vi "PC MAIN.vi"() -> ()   [LabVIEW 2017]
uses:
  <vilib>/Platform/TimedLoop/XDataNode/timing_clust.ctl
  <vilib>/Platform/TimedLoop/XDataNode/nitl_modes.ctl
  <vilib>/Platform/TimedLoop/XDataNode/wakeup.ctl
  <vilib>/imath/engines/lvmath2/RunTimeEngine/IndexRead/NIMS V(S).vi
  <instcachedir>/0/NIMS V(S)_0488751826AF41519A22953C041130DC.lvgen/NIMS V(S)_0488751826AF41519A22953C041130DC_000.vi
  <vilib>/imathl/engines/lvmath/Functions/Error Handling/Create Error.vi
  <vilib>/imath/engines/lvmath2/RunTimeEngine/BuiltInFunctions/atan2/NIMS_atan2.vi
  <instcachedir>/0/NIMS_atan2_A91AA4A7D42247EDBE8F76DB99AF04A4.lvgen/NIMS_atan2_A91AA4A7D42247EDBE8F76DB99AF04A4_000.vi
  <vilib>/imath/engines/lvmath2/RunTimeEngine/IndexReplace/NIMS V(S)=S.vi
  <instcachedir>/0/NIMS V(S)=S_3F4D177D41884A9C969E5FA0B22E4B28.lvgen/NIMS V(S)=S_3F4D177D41884A9C969E5FA0B22E4B28_000.vi
  <vilib>/imath/engines/lvmath2/RunTimeEngine/ArithmeticOperatorToken/NIMS_ArithmeticOperator_power(S).vi
  <instcachedir>/0/NIMS_ArithmeticOperator_power(S)_86B1D76B77564424912EAFCCCC7488ED.lvgen/NIMS_ArithmeticOperator_power(S)_86B1D76B77564424912EAFCCCC7488ED_010.vi
  <vilib>/imath/engines/lvmath2/RunTimeEngine/BuiltInFunctions/acos/NIMS_acos(C).vi
  <instcachedir>/0/NIMS_acos(C)_09AB0EA1D77D44F8AD620F57E6E2841E.lvgen/NIMS_acos(C)_09AB0EA1D77D44F8AD620F57E6E2841E_001.vi
  <instcachedir>/0/NIMS_atan2_A91AA4A7D42247EDBE8F76DB99AF04A4.lvgen/NIMS_atan2_A91AA4A7D42247EDBE8F76DB99AF04A4_001.vi
  <vilib>/imath/engines/lvmath2/RunTimeEngine/BuiltInFunctions/asin/NIMS_asin(C).vi
  <instcachedir>/0/NIMS_asin(C)_AC3BFCB47B1546A49EF59786BF54013C.lvgen/NIMS_asin(C)_AC3BFCB47B1546A49EF59786BF54013C_001.vi
  <instcachedir>/0/NIMS V(S)=S_3F4D177D41884A9C969E5FA0B22E4B28.lvgen/NIMS V(S)=S_3F4D177D41884A9C969E5FA0B22E4B28_001.vi
  <vilib>/imath/engines/lvmath2/RunTimeEngine/ErrorHandling/NIMS_Create Error From Enums.vi
  <instcachedir>/0/NIMS V(S)_0488751826AF41519A22953C041130DC.lvgen/NIMS V(S)_0488751826AF41519A22953C041130DC_003.vi
  <vilib>/imath/engines/lvmath2/RunTimeEngine/BuiltInFunctions/sin/NIMS_sin(C).vi
  <instcachedir>/0/NIMS_sin(C)_3AEF00A0D47841AA8A3F5FC7392BEEFD.lvgen/NIMS_sin(C)_3AEF00A0D47841AA8A3F5FC7392BEEFD_001.vi
  <vilib>/imath/engines/lvmath2/RunTimeEngine/BuiltInFunctions/cos/NIMS_cos(C).vi
  <instcachedir>/0/NIMS_cos(C)_D76AB42705D04DD7AB90183D51B32C21.lvgen/NIMS_cos(C)_D76AB42705D04DD7AB90183D51B32C21_001.vi
  <vilib>/imath/engines/lvmath2/RunTimeEngine/BuiltInFunctions/pinv/NIMS_pinv.vi
  <instcachedir>/0/NIMS_pinv_206F0700CF75499C820074BA4F1FFC36.lvgen/NIMS_pinv_206F0700CF75499C820074BA4F1FFC36_001.vi
  <vilib>/imath/engines/lvmath2/RunTimeEngine/ArithmeticOperatorToken/NIMS_ArithmeticOperator_multmx(M,CV).vi
  <instcachedir>/0/NIMS_ArithmeticOperator_multmx(M,CV)_C4CEBAC88ACD4FCE9121CEED56911FC5.lvgen/NIMS_ArithmeticOperator_multmx(M,CV)_C4CEBAC88ACD4FCE9121CEED56911FC5_002.vi
  <vilib>/imath/engines/lvmath2/RunTimeEngine/IndexRead/NIMS M($,S).vi
  <instcachedir>/0/NIMS M($,S)_3E5749BBB62E49528D4765A77F1F6D98.lvgen/NIMS M($,S)_3E5749BBB62E49528D4765A77F1F6D98_001.vi
  <vilib>/imath/engines/lvmath2/RunTimeEngine/NodeEndStatement/NIMS_NodeEndStatement_Output.vi
  <instcachedir>/0/NIMS_NodeEndStatement_Output_53EC0D466D134D7ABD903AC30B43404B.lvgen/NIMS_NodeEndStatement_Output_53EC0D466D134D7ABD903AC30B43404B_000.vi
  <vilib>/imath/engines/lvmath2/RunTimeEngine/ErrorHandling/NIMS_Finalize Error.vi
  <vilib>/imath/engines/lvmath2/RunTimeEngine/RangeToken/NIMS_Range_R2 - Integer.vi
  <instcachedir>/0/NIMS_Range_R2 - Integer_B2C3C6B11D0E4F789E1772ACB483EB02.lvgen/NIMS_Range_R2 - Integer_B2C3C6B11D0E4F789E1772ACB483EB02_000.vi
  <vilib>/imath/engines/lvmath2/RunTimeEngine/CommandStatement/MC_CommandStatement_break.vi
  <vilib>/imath/engines/lvmath2/RunTimeEngine/VariableToken/NIMS_VariableToken_CondDefinedDefinedByReplace.vi
  <instcachedir>/0/NIMS_VariableToken_CondDefinedDefinedByReplace_D162CFFC24174562A9FEA619A91E1A56.lvgen/NIMS_VariableToken_CondDefinedDefinedByReplace_D162CFFC24174562A9FEA619A91E1A56_000.vi
  <instcachedir>/0/NIMS_VariableToken_CondDefinedDefinedByReplace_D162CFFC24174562A9FEA619A91E1A56.lvgen/NIMS_VariableToken_CondDefinedDefinedByReplace_D162CFFC24174562A9FEA619A91E1A56_003.vi
  <instcachedir>/0/NIMS_VariableToken_CondDefinedDefinedByReplace_D162CFFC24174562A9FEA619A91E1A56.lvgen/NIMS_VariableToken_CondDefinedDefinedByReplace_D162CFFC24174562A9FEA619A91E1A56_002.vi
  <vilib>/imath/engines/lvmath2/RunTimeEngine/VariableToken/NIMS_VariableToken_CondDefined.vi
  <instcachedir>/0/NIMS_VariableToken_CondDefined_6E7F1EE7F80E48298C84CF05BD736261.lvgen/NIMS_VariableToken_CondDefined_6E7F1EE7F80E48298C84CF05BD736261_000.vi
  <vilib>/imath/engines/lvmath2/RunTimeEngine/IndexReplace/NIMS M(S,S)=S.vi
  <instcachedir>/0/NIMS M(S,S)=S_490F2BBDD0204024B81939EC402D9A55.lvgen/NIMS M(S,S)=S_490F2BBDD0204024B81939EC402D9A55_001.vi
  <instcachedir>/0/NIMS_VariableToken_CondDefined_6E7F1EE7F80E48298C84CF05BD736261.lvgen/NIMS_VariableToken_CondDefined_6E7F1EE7F80E48298C84CF05BD736261_002.vi
  <instcachedir>/0/NIMS_NodeEndStatement_Output_53EC0D466D134D7ABD903AC30B43404B.lvgen/NIMS_NodeEndStatement_Output_53EC0D466D134D7ABD903AC30B43404B_003.vi
  <vilib>/platform/TimedLoop/XDataNode/XDataNode.xnode
  <vilib>/Platform/TimedLoop/XDataNode/XDNodeRunTimeDep.lvlib
panel:
  in  "Z-":bool
  in  "Z+":bool
  in  "Y-":bool
  in  "Y+":bool
  in  "X-":bool
  out "x":dbl[][](array[numeric])
  in  "Increment(0-10mm)":dbl min=-10.0 max=10.0 step=1.0
  in  "X+":bool
  out "Joint3":dbl
  out "Joint2":dbl
  out "Joint1":dbl
  in  "Circle":bool
  out "circle":dbl[](array[numeric])
  out "line":dbl[](array[numeric])
  in  "Line":bool
  in  "DIR3":bool
  in  "Duty cycle3":dbl
  in  "Frequency3":dbl
  in  "DIR2":bool
  in  "Duty cycle2":dbl
  in  "Frequency2":dbl
  in  "RT STOP":bool
  in  "DIR1":bool
  in  "Duty cycle1":dbl
  in  "Frequency1":dbl
  in  "STOP":bool
  # "Motor Status"
  # "Control Pad"
  # "Joint Angle(Deg)"
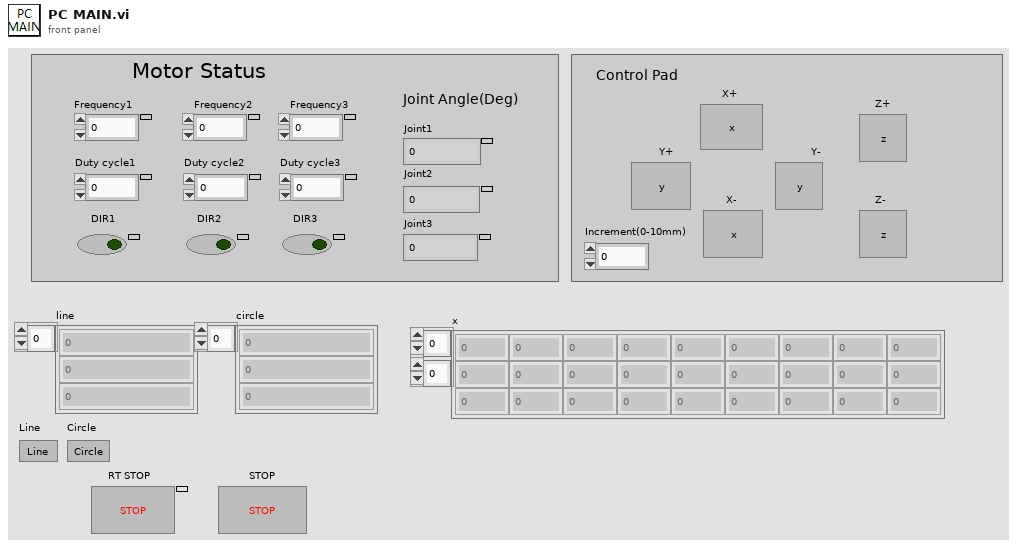
[diagram p1: front panel]
types:
  T1 = typedef "XDNodeRunTimeDep.lvlib/timing_clust.ctl" = cluster{"Expected End [f-1]":u64, "Actual End [f-1]":u64, "Finished Late? [f-1]":bool, "Expected End [i-1]":u64, "Actual End [i-1]":u64, "Finished Late? [i-1]":bool, "Expected Start [i]":u64, "Actual Start [i]":u64, "Expected Start [f]":u64, "Actual Start [f]":u64, "Source Name":string, "Structure Name":string, "Period":i64, "Deadline":i64, "Offset":i64, "Start":i64, "Priority":i32, "Timeout":i32, "Mode":T2, "Wakeup Reason":T3, "Error":errorcluster, "Source Type":string, "Secondary Source Type":string, "Global End Time":u64, "Global Start Time":u64, "Frame Duration":u64, "Iteration Duration":u64, "Assigned CPU":i32, "I/O Scan Engine Mode":u32}
  T2 = typedef "XDNodeRunTimeDep.lvlib/nitl_modes.ctl" = enum32{"No Change", "Process missed periods, maintain original phase", "Discard missed periods, maintain original phase", "Process missed periods, ignore original phase", "Discard missed periods, ignore original phase"}
  T3 = typedef "XDNodeRunTimeDep.lvlib/wakeup.ctl" = enum32{"Normal", "Aborted", "Asynchronous wakeup", "Timing source error", "Timed loop error", "Timeout"}
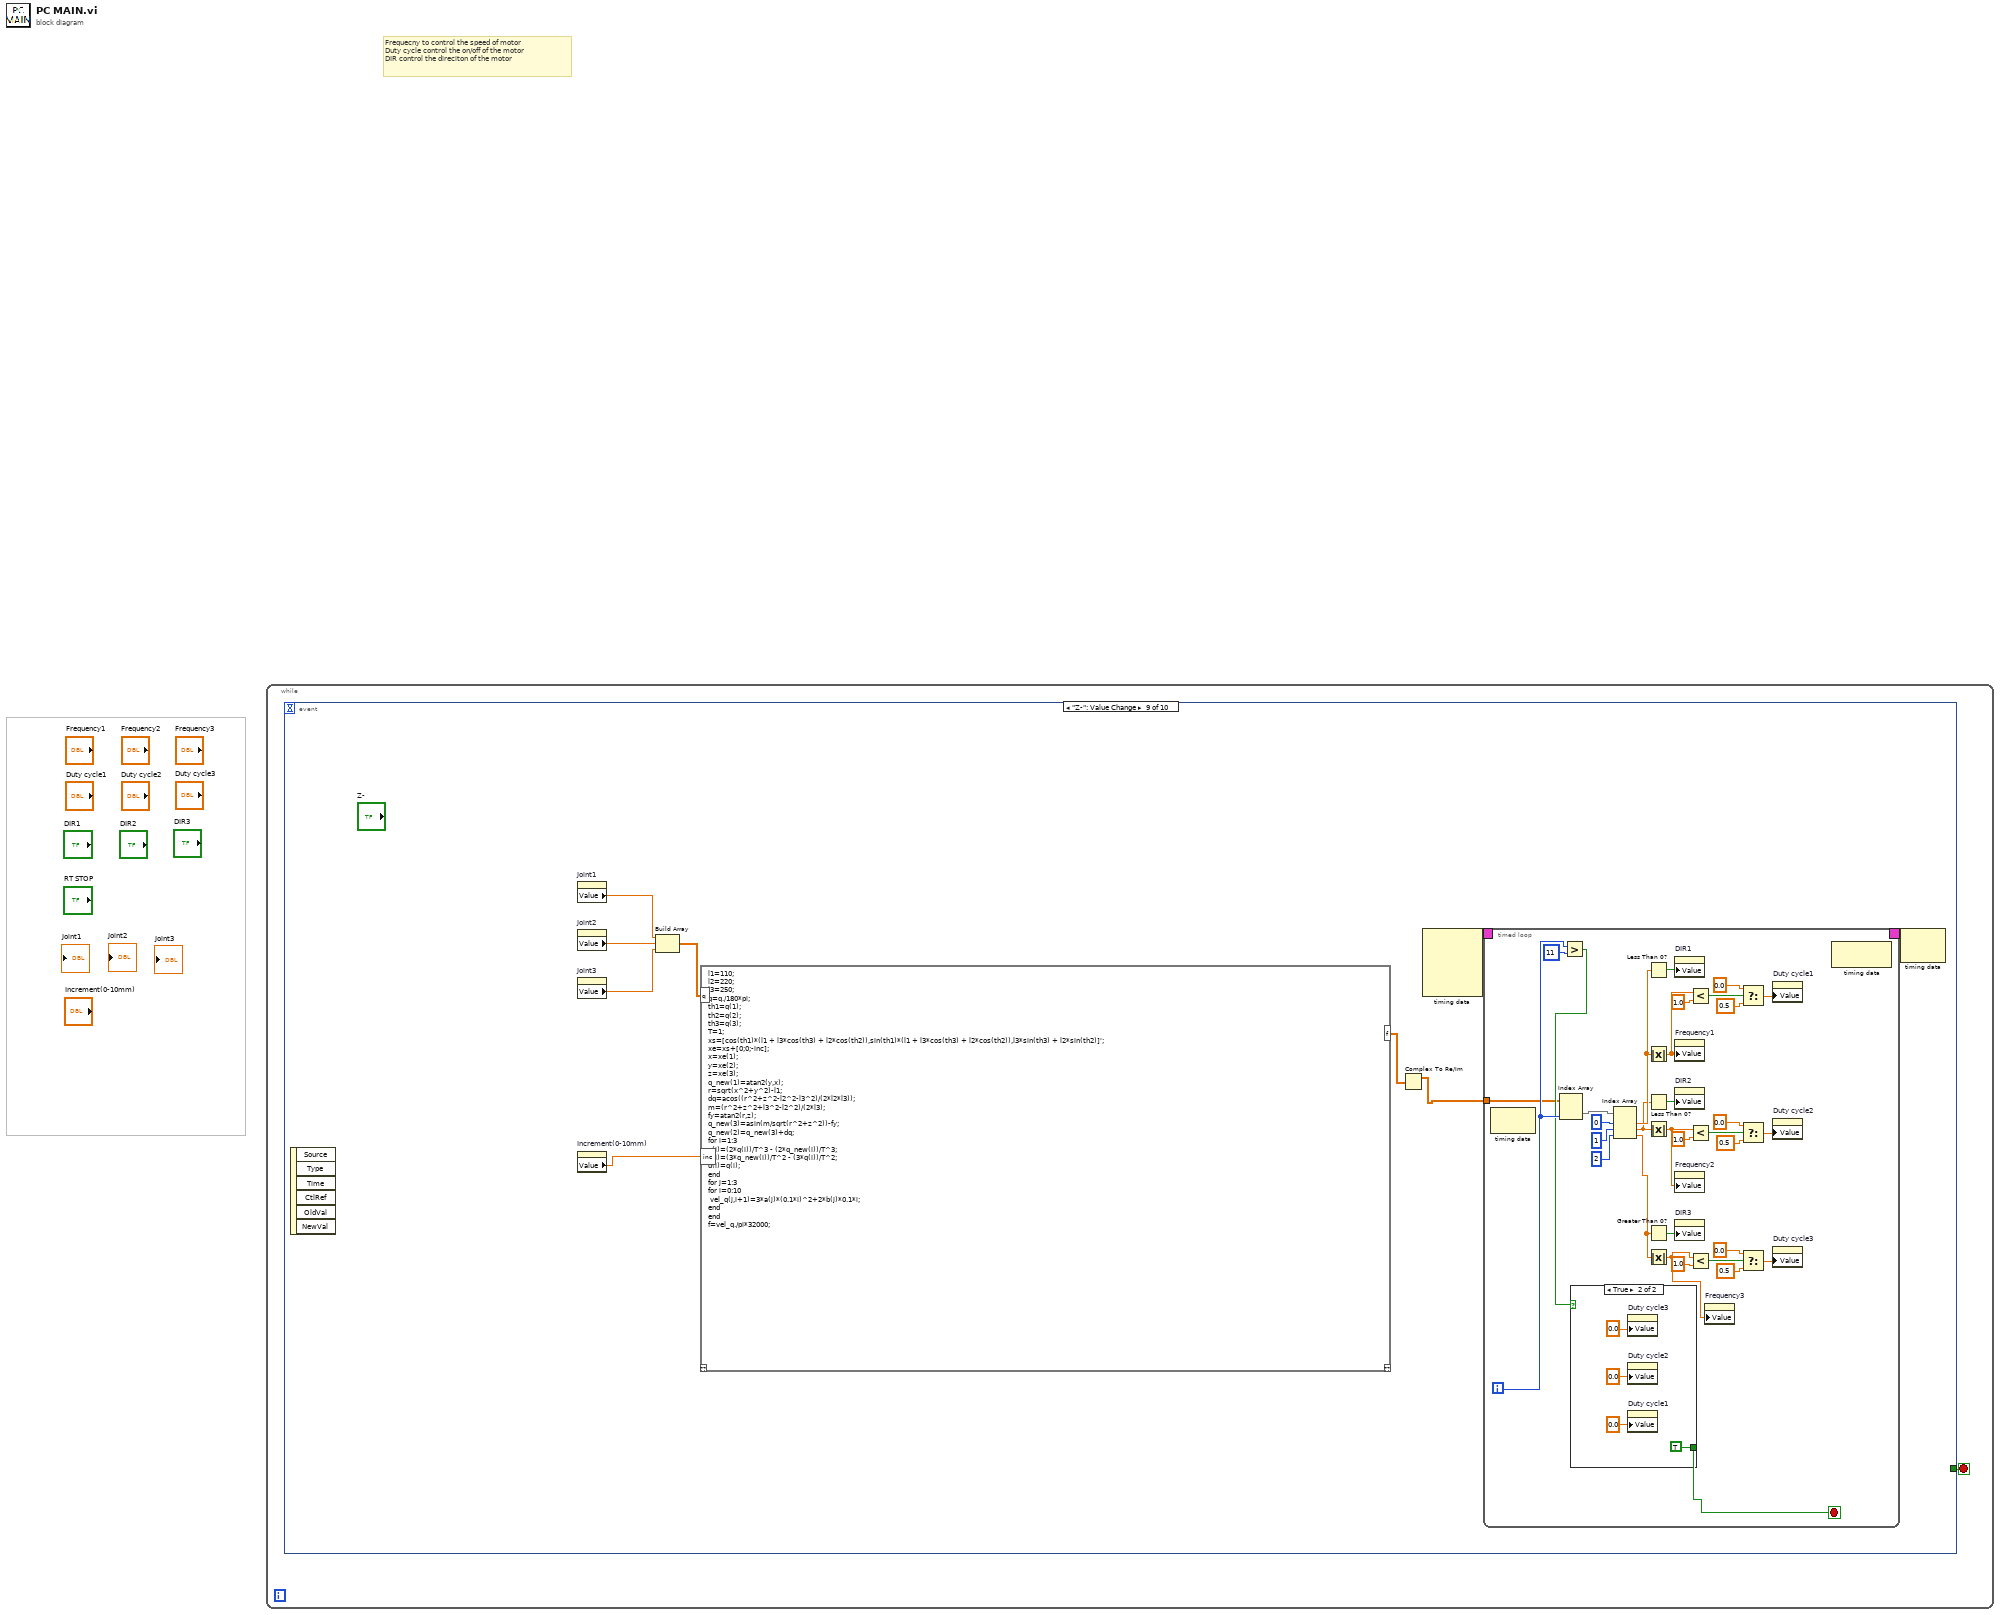
[diagram p0: block diagram]
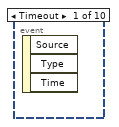
[diagram p2: hidden frame]
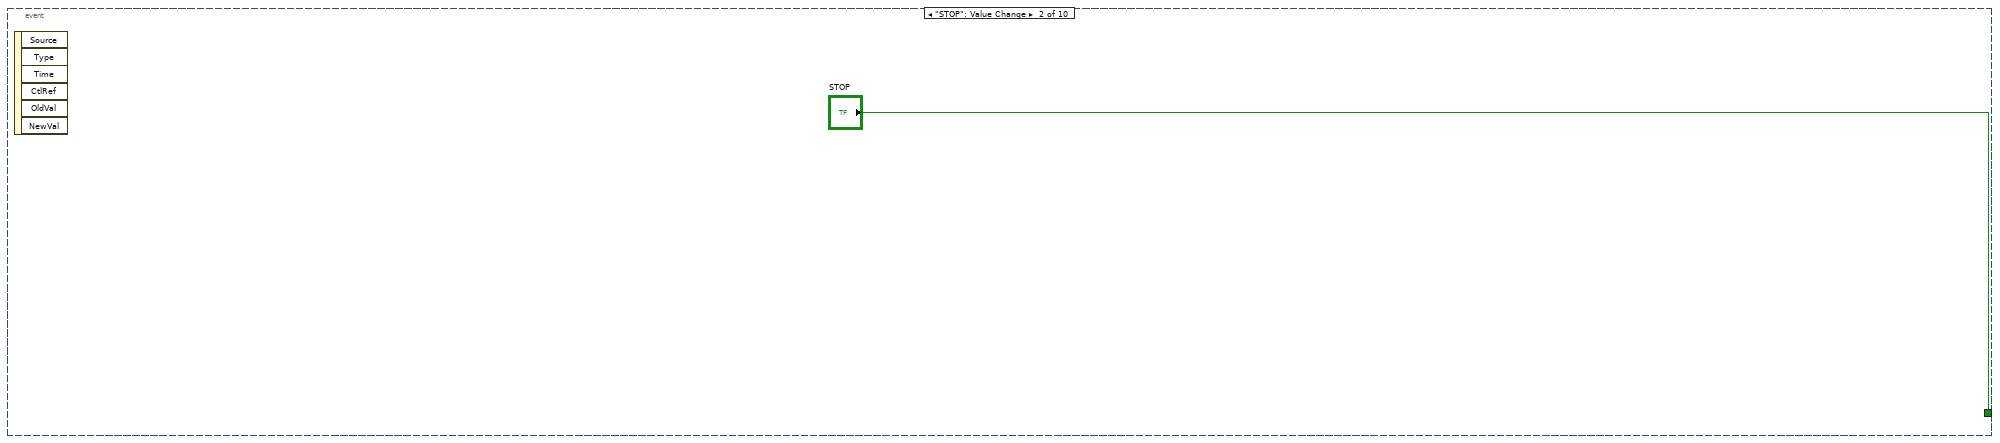
[diagram p3: hidden frame]
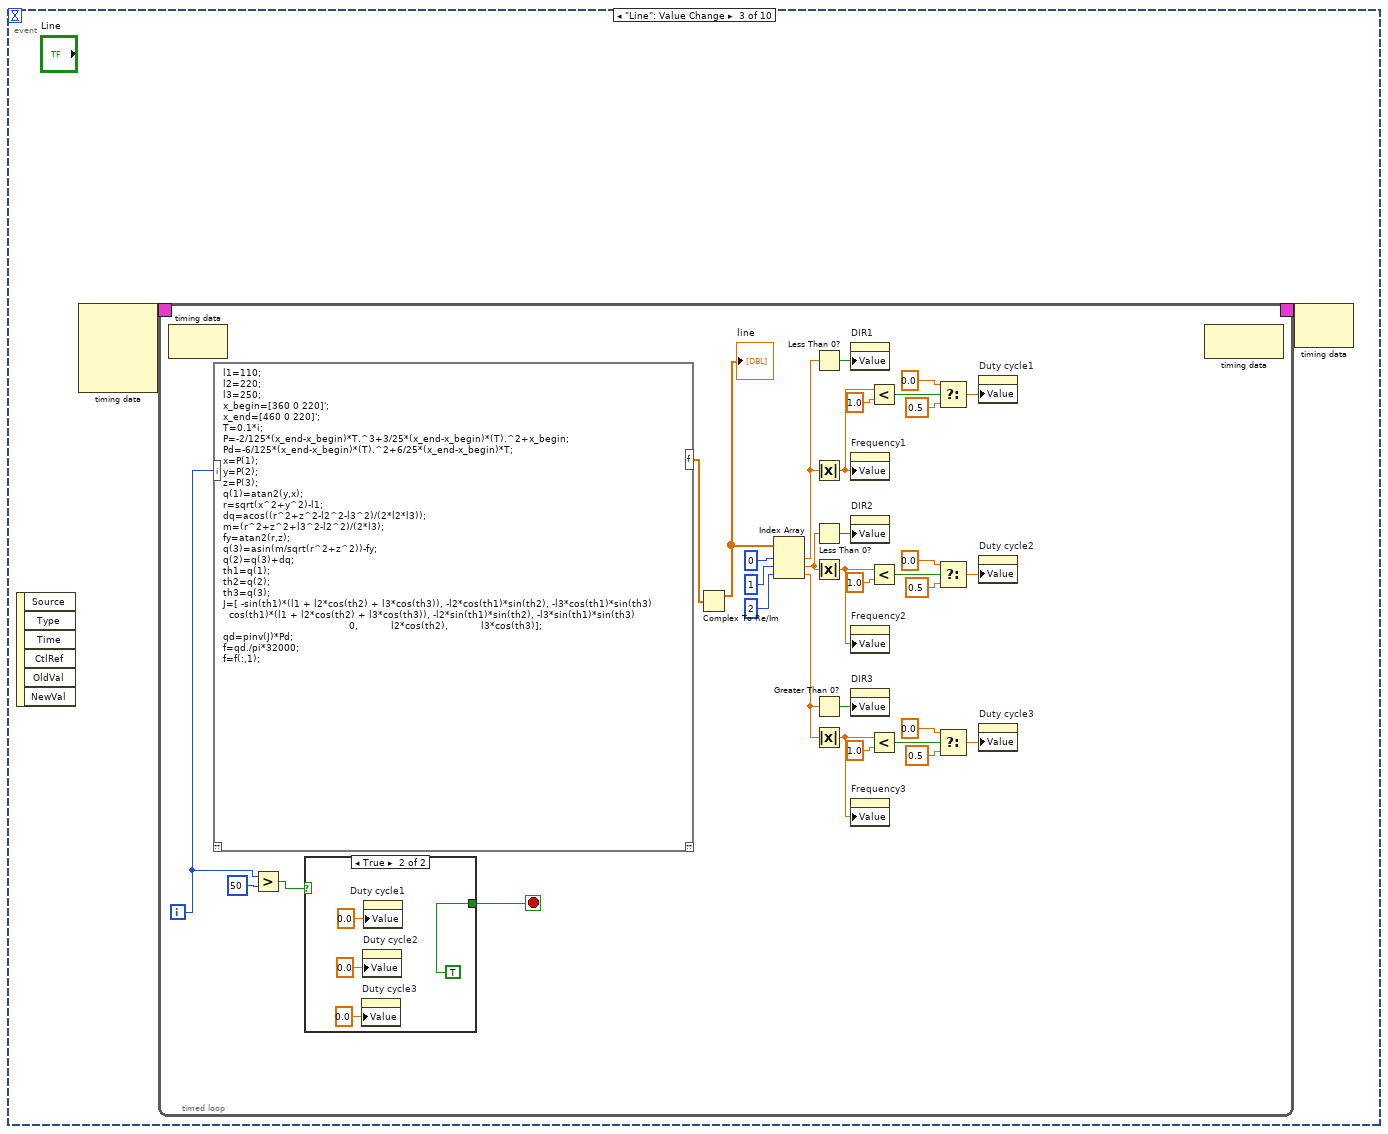
[diagram p4: hidden frame]
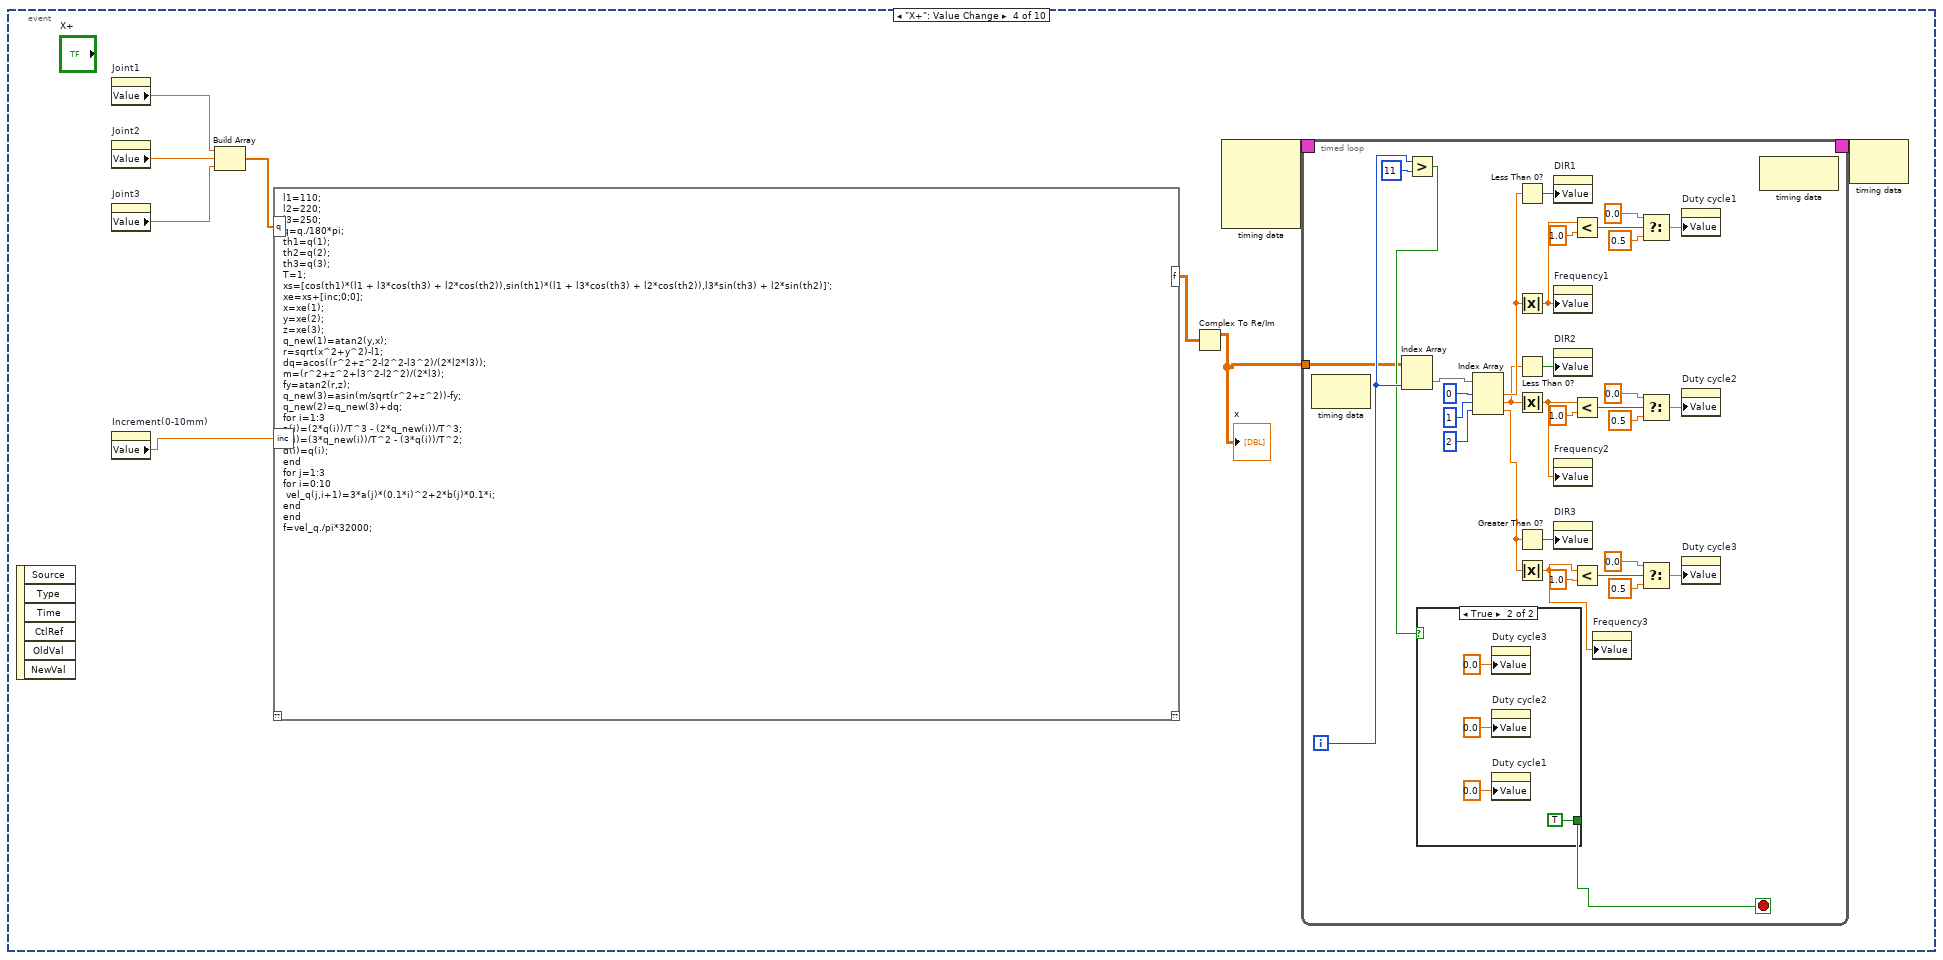
[diagram p6: hidden frame]
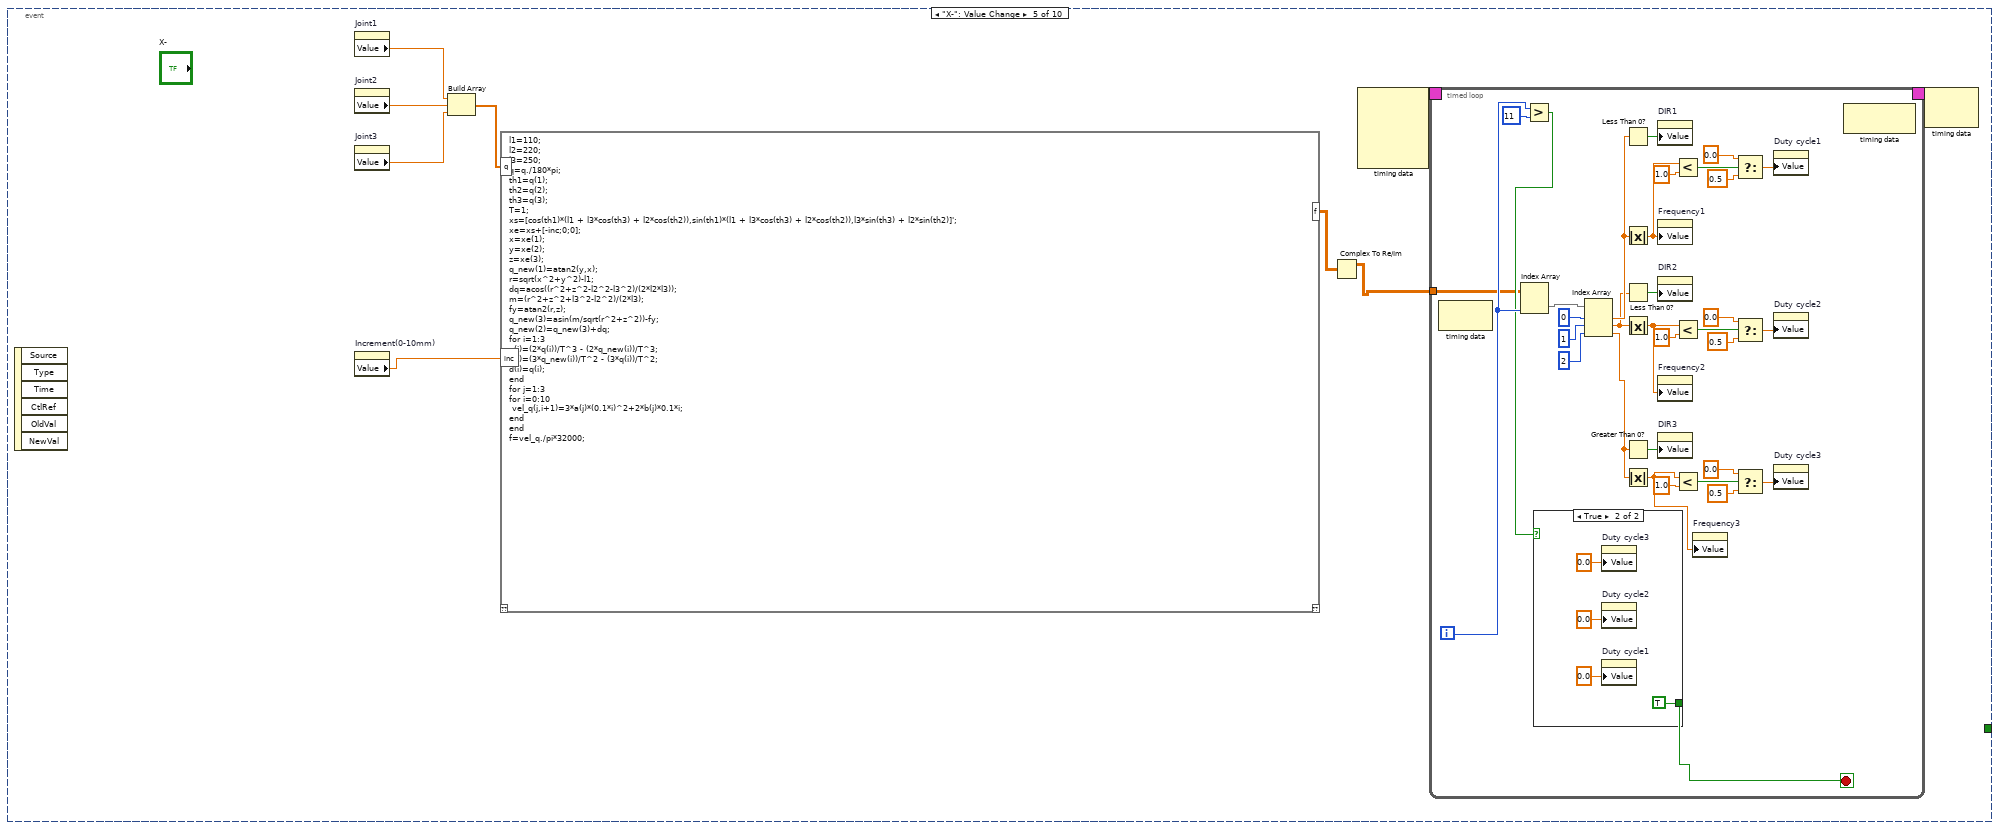
[diagram p8: hidden frame]
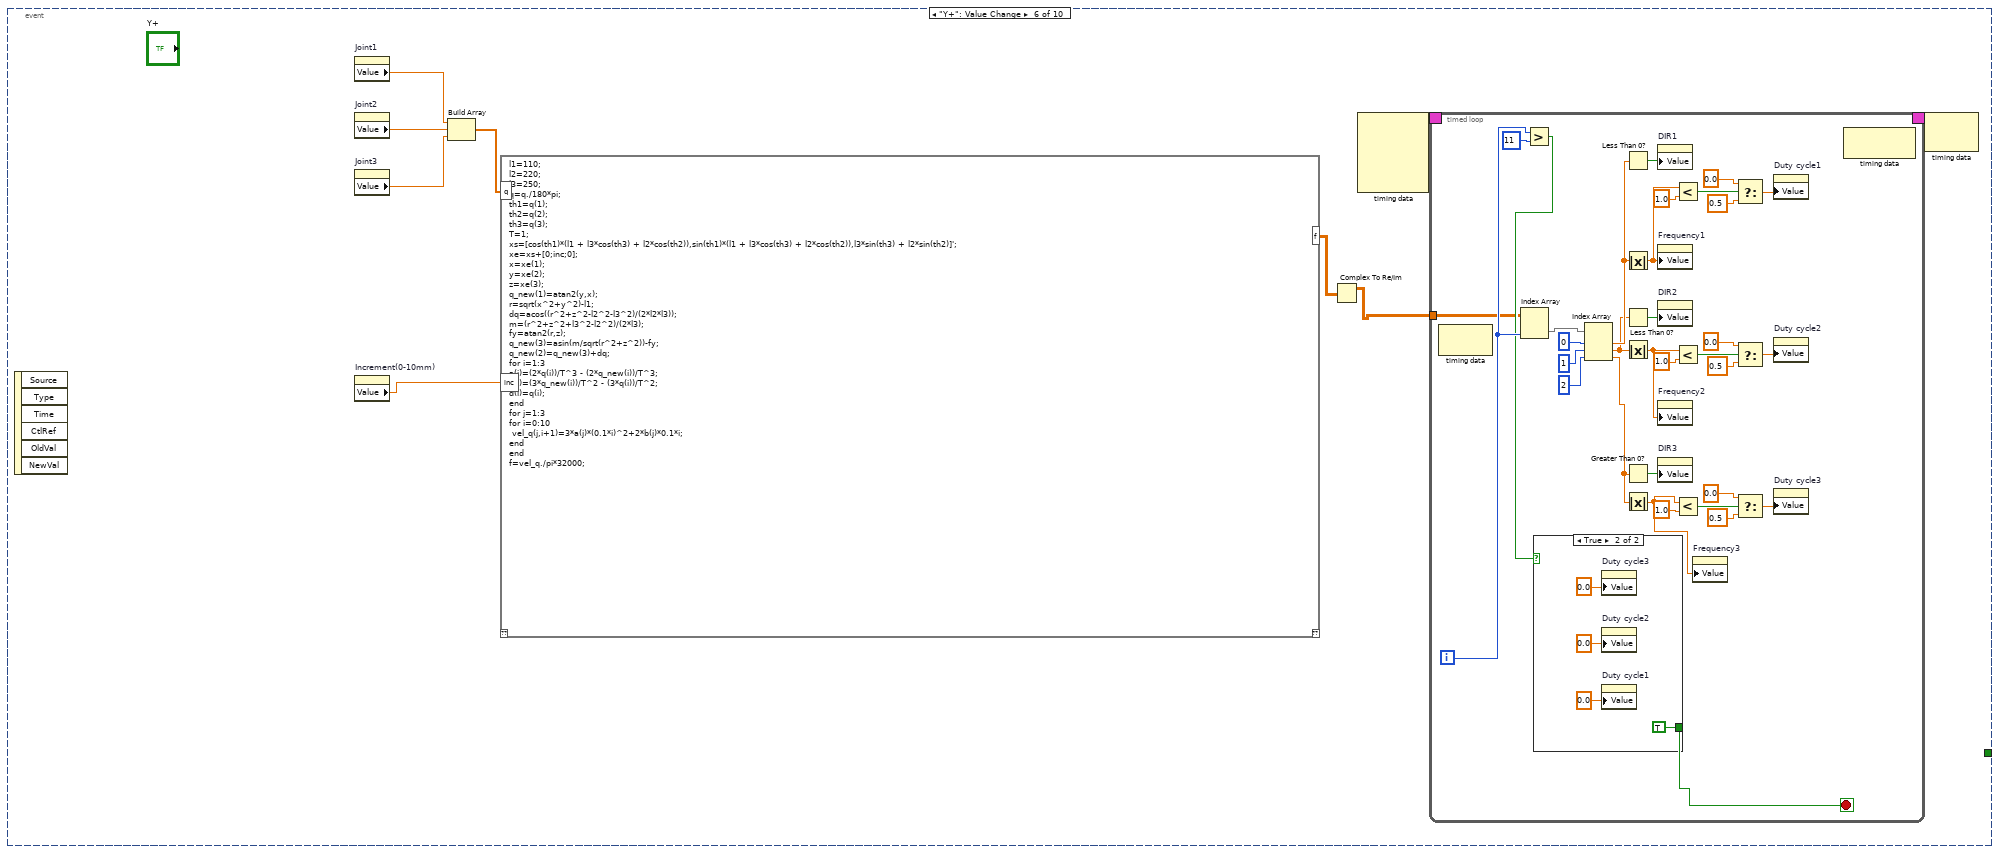
[diagram p10: hidden frame]
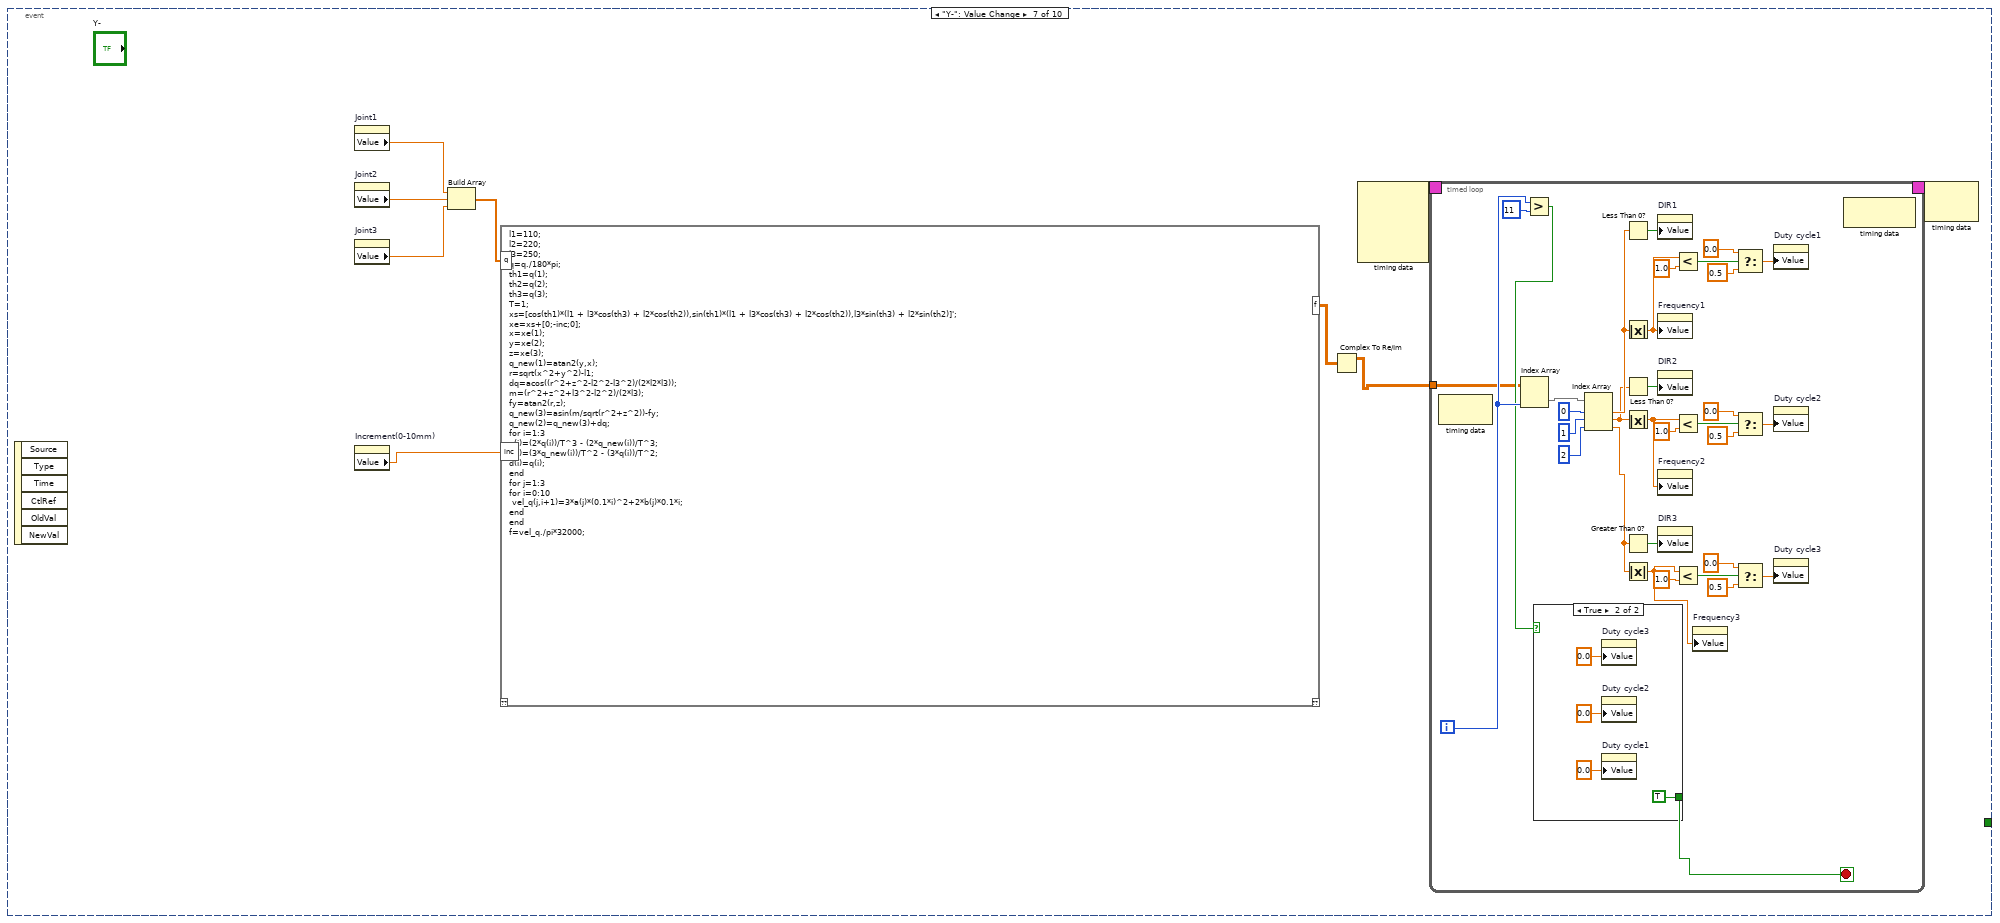
[diagram p12: hidden frame]
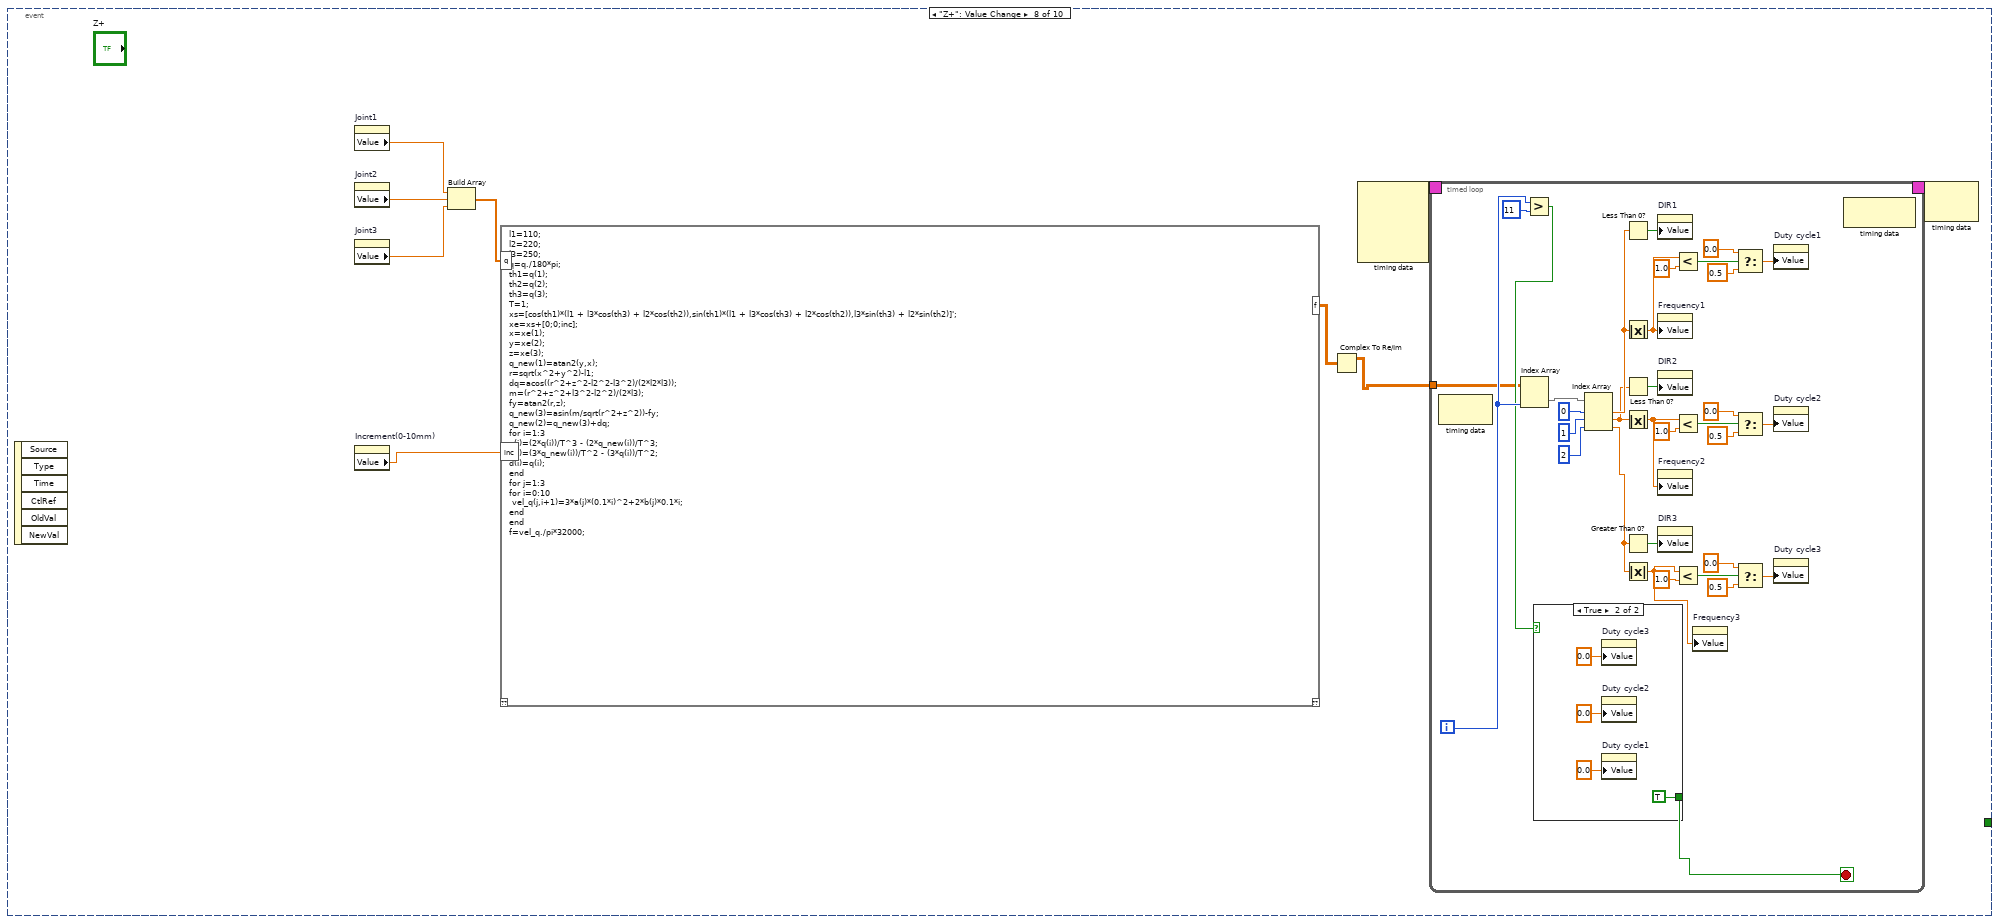
[diagram p14: hidden frame]
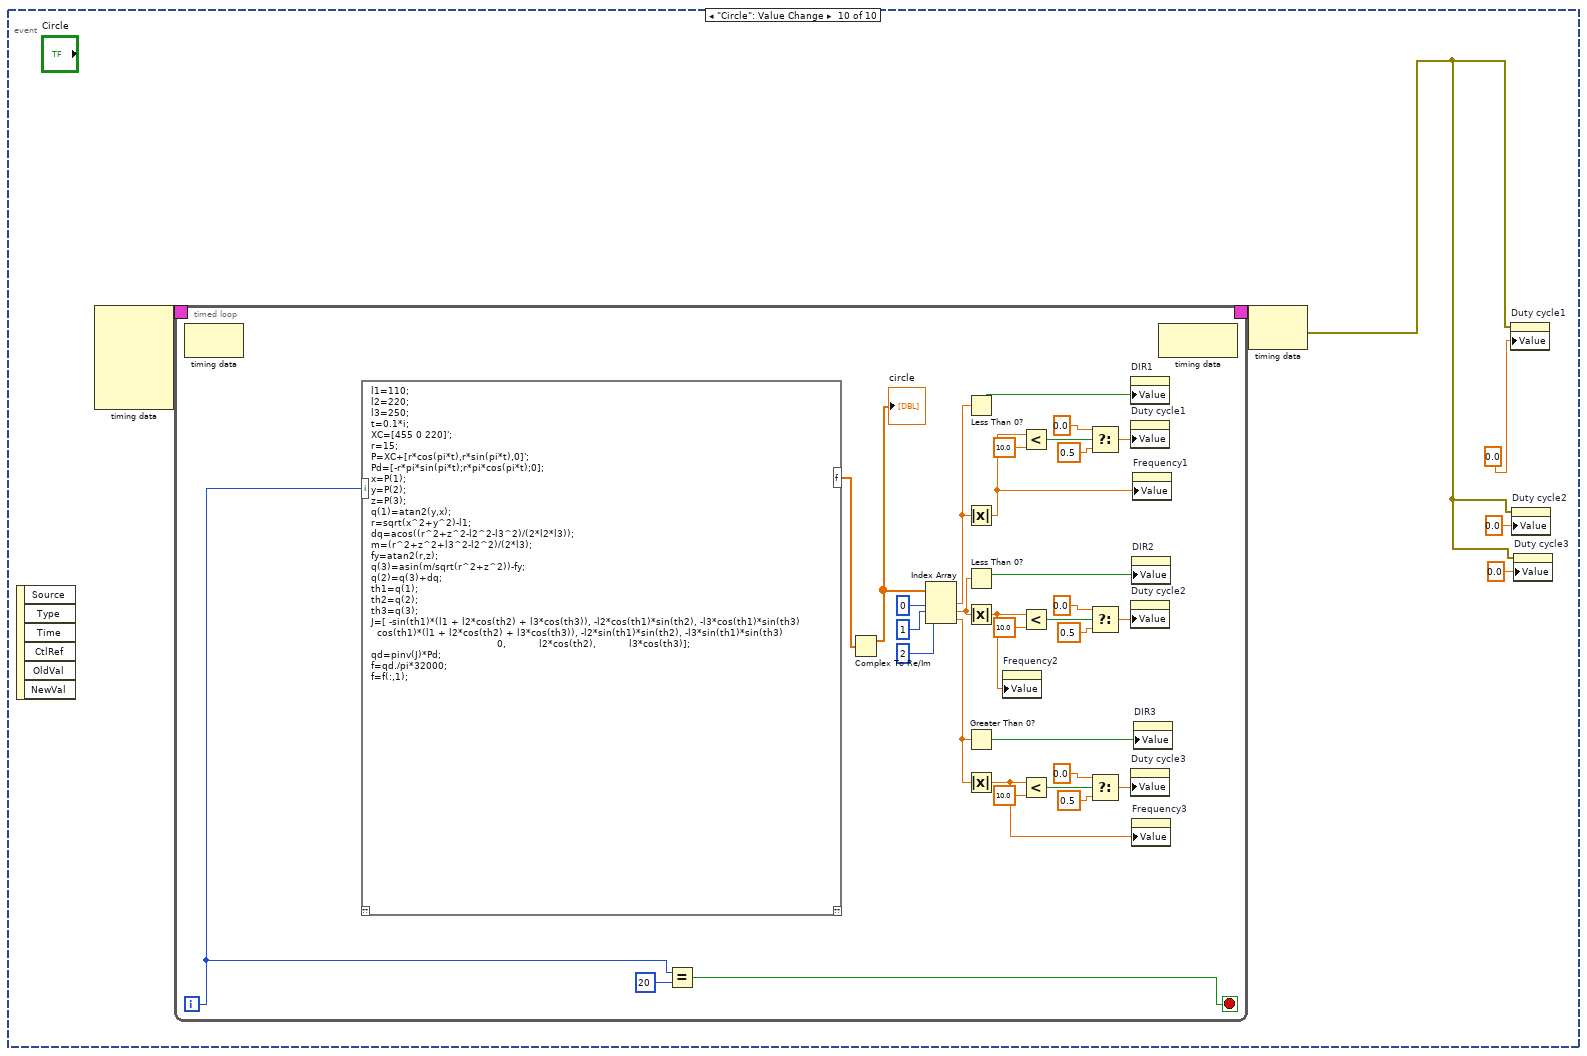
[diagram p17: hidden frame]
diagram:
  # "Frequecny to control the speed of motor \nDuty cycle control the on/off of the motor\nDIR control the direciton of the motor"
  n1 = while {
    stop <- w1 stop-if-true
    n2 = event shown="[8] \"Z-\": Value Change" {
      selector: _ -> [_ _ _ _ _ _ _ _ _ _]
      dyn-events: _ -> [_ _ _ _ _ _ _ _ _ _]
      timeout: _ -> [_ _ _ _ _ _ _ _ _ _]
      tunnel: [_ "STOP" _ _ _ _ _ _ _ _] -> w1
      event Timeout {
        n3 = event-data() -> ()  [unwired: 1 in, 3 out]
      }
      event "STOP": Value Change {
        n4 = event-data() -> ()  [unwired: 1 in, 6 out]
      }
      event "Line": Value Change {
        n5 = event-data() -> ()  [unwired: 1 in, 6 out]
        n6 = node-c288() -> (w4:T1)  [unwired: 4 in]
        n7 = timed-loop {
          timing: w4 -> [_]
          timing-out: [_] -> w3
          i -> [w37]
          stop <- w5 stop-if-true
          n8 = node-c288() -> ()  [unwired: 1 in, 1 out]
          n9 = mathscript code="l1=110;\nl2=220;\nl3=250;\nx_begin=[360 0 220]';\nx_end=[460 0 220]';\nT=0.1*i;\nP=-2/125*(x_end-x_begin)*T.^3+3/25*(x_end-x_begin)*(T).^2+x_begin;\nPd=-6/125*(x_end-x_begin)*(T).^2+6/25*(x_end-x_begin)*T;\nx=P(1);\ny=P(2);\nz=P(3);\nq(1)=atan2(y,x);\nr=sqrt(x^2+y^2)-l1;\ndq=acos((r^2+z^2-l2^2-l3^2)/(2*l2*l3));\nm=(r^2+z^2+l3^2-l2^2)/(2*l3);\nfy=atan2(r,z);\nq(3)=asin(m/sqrt(r^2+z^2))-fy;\nq(2)=q(3)+dq;\nth1=q(1);\nth2=q(2);\nth3=q(3);\nJ=[ -sin(th1)*(l1 + l2*cos(th2) + l3*cos(th3)), -l2*cos(th1)*sin(th2), -l3*cos(th1)*sin(th3)\n  cos(th1)*(l1 + l2*cos(th2) + l3*cos(th3)), -l2*sin(th1)*sin(th2), -l3*sin(th1)*sin(th3)\n                                          0,           l2*cos(th2),           l3*cos(th3)];\nqd=pinv(J)*Pd;\nf=qd./pi*32000;\nf=f(:,1);"("i"=w37) -> ("f"=w35:cdb[])  [unwired: 1 in, 1 out]
          n10 = Greater?(x=w37, y=50) -> (0:w6:bool)
          n11 = case shown="True" w6 {
            tunnel: [_ TRUE] -> w5
            frame False {
            }
            frame True {
              n12 = property on="Duty cycle3" class="DigNum (strict)"("Value"=0.0 ("Duty cycle3")) -> ()  [unwired: 2 in, 2 out]
              n13 = property on="Duty cycle2" class="DigNum (strict)"("Value"=0.0 ("Duty cycle2")) -> ()  [unwired: 2 in, 2 out]
              n14 = property on="Duty cycle1" class="DigNum (strict)"("Value"=0.0 ("Duty cycle1")) -> ()  [unwired: 2 in, 2 out]
            }
          }
          n15 = Complex To Re/Im(x + iy=w35) -> (x=w34:dbl[])  [unwired: 1 out]
          "line" <- w34
          n16 = Index Array(array=w34, index #1=0 ("index"), index #2=1 ("index"), index #3=2 ("index")) -> (element #1=w29:dbl, element #2=w20:dbl, element #3=w19:dbl)
          n17 = Less Than 0?(x=w29) -> (x < 0?=w30:bool)
          n18 = Absolute Value(x=w29) -> (abs(x)=w18:dbl)
          n19 = Less Than 0?(x=w20) -> (x < 0?=w28:bool)
          n20 = Absolute Value(x=w20) -> (abs(x)=w12:dbl)
          n21 = Greater Than 0?(x=w19) -> (x > 0?=w21:bool)
          n22 = Absolute Value(x=w19) -> (abs(x)=w9:dbl)
          n23 = property on="DIR1" class="Bool (strict)"("Value"=w30) -> ()  [unwired: 2 in, 2 out]
          n24 = property on="Frequency1" class="DigNum (strict)"("Value"=w18) -> ()  [unwired: 2 in, 2 out]
          n25 = property on="DIR2" class="Bool (strict)"("Value"=w28) -> ()  [unwired: 2 in, 2 out]
          n26 = property on="Frequency2" class="DigNum (strict)"("Value"=w12) -> ()  [unwired: 2 in, 2 out]
          n27 = property on="DIR3" class="Bool (strict)"("Value"=w21) -> ()  [unwired: 2 in, 2 out]
          n28 = property on="Frequency3" class="DigNum (strict)"("Value"=w9) -> ()  [unwired: 2 in, 2 out]
          n29 = Less?(x=w18, y=1.0) -> (x < y?=w16:bool)
          n30 = Less?(x=w12, y=1.0) -> (x < y?=w10:bool)
          n31 = Less?(x=w9, y=1.0) -> (x < y?=w7:bool)
          n32 = Select(t=0.0, s=w16, f=0.5) -> (s? t:f=w13:dbl)
          n33 = Select(t=0.0, s=w10, f=0.5) -> (s? t:f=w27:dbl)
          n34 = Select(t=0.0, s=w7, f=0.5) -> (s? t:f=w22:dbl)
          n35 = property on="Duty cycle1" class="DigNum (strict)"("Value"=w13) -> ()  [unwired: 2 in, 2 out]
          n36 = property on="Duty cycle2" class="DigNum (strict)"("Value"=w27) -> ()  [unwired: 2 in, 2 out]
          n37 = property on="Duty cycle3" class="DigNum (strict)"("Value"=w22) -> ()  [unwired: 2 in, 2 out]
          n38 = node-c288() -> ()  [unwired: 1 in, 1 out]
        }
        n39 = node-c288(w3) -> ()  [unwired: 1 out]
      }
      event "X+": Value Change {
        n40 = event-data() -> ()  [unwired: 1 in, 6 out]
        n41 = property on="Joint1" class="DigNum (strict)"() -> ("Value"=w563:dbl)  [unwired: 2 in, 2 out]
        n42 = property on="Joint2" class="DigNum (strict)"() -> ("Value"=w562:dbl)  [unwired: 2 in, 2 out]
        n43 = property on="Joint3" class="DigNum (strict)"() -> ("Value"=w561:dbl)  [unwired: 2 in, 2 out]
        n44 = property on="Increment(0-10mm)" class="DigNum (strict)"() -> ("Value"=w557:dbl)  [unwired: 2 in, 2 out]
        n45 = Build Array(w563, w562, w561) -> (w560:dbl[])
        n46 = mathscript code="l1=110;\nl2=220;\nl3=250;\nq=q./180*pi;\nth1=q(1);\nth2=q(2);\nth3=q(3);\nT=1;\nxs=[cos(th1)*(l1 + l3*cos(th3) + l2*cos(th2)),sin(th1)*(l1 + l3*cos(th3) + l2*cos(th2)),l3*sin(th3) + l2*sin(th2)]';\nxe=xs+[inc;0;0];\nx=xe(1);\ny=xe(2);\nz=xe(3);\nq_new(1)=atan2(y,x);\nr=sqrt(x^2+y^2)-l1;\ndq=acos((r^2+z^2-l2^2-l3^2)/(2*l2*l3));\nm=(r^2+z^2+l3^2-l2^2)/(2*l3);\nfy=atan2(r,z);\nq_new(3)=asin(m/sqrt(r^2+z^2))-fy;\nq_new(2)=q_new(3)+dq;\nfor i=1:3\na(i)=(2*q(i))/T^3 - (2*q_new(i))/T^3;\nb(i)=(3*q_new(i))/T^2 - (3*q(i))/T^2;\nd(i)=q(i);\nend\nfor j=1:3\nfor i=0:10\n vel_q(j,i+1)=3*a(j)*(0.1*i)^2+2*b(j)*0.1*i;\nend\nend\nf=vel_q./pi*32000;"("q"=w560, "inc"=w557) -> ("f"=w556:cdb[][])  [unwired: 1 in, 1 out]
        n47 = Complex To Re/Im(x + iy=w556) -> (x=w555:dbl[][])  [unwired: 1 out]
        "x" <- w555
        n48 = node-c288() -> (w559:T1)  [unwired: 4 in]
        n49 = timed-loop {
          timing: w559 -> [_]
          timing-out: [_] -> w558
          tunnel: w555 -> [w568]
          i -> [w572]
          stop <- w569 stop-if-true
          n50 = node-c288() -> ()  [unwired: 1 in, 1 out]
          n51 = Index Array(array=w568, index (col)=w572) -> (element=w567:dbl[])  [unwired: 1 in]
          n52 = Greater?(x=w572, y=11) -> (0:w570:bool)
          n53 = case shown="True" w570 {
            tunnel: [_ TRUE] -> w569
            frame False {
            }
            frame True {
              n54 = property on="Duty cycle3" class="DigNum (strict)"("Value"=0.0 ("Duty cycle3")) -> ()  [unwired: 2 in, 2 out]
              n55 = property on="Duty cycle2" class="DigNum (strict)"("Value"=0.0 ("Duty cycle2")) -> ()  [unwired: 2 in, 2 out]
              n56 = property on="Duty cycle1" class="DigNum (strict)"("Value"=0.0 ("Duty cycle1")) -> ()  [unwired: 2 in, 2 out]
            }
          }
          n57 = Index Array(array=w567, index #1=0 ("index"), index #2=1 ("index"), index #3=2 ("index")) -> (element #1=w566:dbl, element #2=w565:dbl, element #3=w564:dbl)
          n58 = Less Than 0?(x=w566) -> (x < 0?=w593:bool)
          n59 = Absolute Value(x=w566) -> (abs(x)=w584:dbl)
          n60 = Less Than 0?(x=w565) -> (x < 0?=w592:bool)
          n61 = Absolute Value(x=w565) -> (abs(x)=w578:dbl)
          n62 = Greater Than 0?(x=w564) -> (x > 0?=w585:bool)
          n63 = Absolute Value(x=w564) -> (abs(x)=w575:dbl)
          n64 = property on="DIR1" class="Bool (strict)"("Value"=w593) -> ()  [unwired: 2 in, 2 out]
          n65 = property on="Frequency1" class="DigNum (strict)"("Value"=w584) -> ()  [unwired: 2 in, 2 out]
          n66 = property on="DIR2" class="Bool (strict)"("Value"=w592) -> ()  [unwired: 2 in, 2 out]
          n67 = property on="Frequency2" class="DigNum (strict)"("Value"=w578) -> ()  [unwired: 2 in, 2 out]
          n68 = property on="DIR3" class="Bool (strict)"("Value"=w585) -> ()  [unwired: 2 in, 2 out]
          n69 = Less?(x=w584, y=1.0) -> (x < y?=w582:bool)
          n70 = Less?(x=w578, y=1.0) -> (x < y?=w576:bool)
          n71 = Less?(x=w575, y=1.0) -> (x < y?=w573:bool)
          n72 = property on="Frequency3" class="DigNum (strict)"("Value"=w575) -> ()  [unwired: 2 in, 2 out]
          n73 = Select(t=0.0, s=w582, f=0.5) -> (s? t:f=w579:dbl)
          n74 = Select(t=0.0, s=w576, f=0.5) -> (s? t:f=w591:dbl)
          n75 = Select(t=0.0, s=w573, f=0.5) -> (s? t:f=w586:dbl)
          n76 = property on="Duty cycle1" class="DigNum (strict)"("Value"=w579) -> ()  [unwired: 2 in, 2 out]
          n77 = property on="Duty cycle2" class="DigNum (strict)"("Value"=w591) -> ()  [unwired: 2 in, 2 out]
          n78 = property on="Duty cycle3" class="DigNum (strict)"("Value"=w586) -> ()  [unwired: 2 in, 2 out]
          n79 = node-c288() -> ()  [unwired: 1 in, 1 out]
        }
        n80 = node-c288(w558) -> ()  [unwired: 1 out]
      }
      event "X-": Value Change {
        n81 = event-data() -> ()  [unwired: 1 in, 6 out]
        n82 = property on="Joint1" class="DigNum (strict)"() -> ("Value"=w1331:dbl)  [unwired: 2 in, 2 out]
        n83 = property on="Joint2" class="DigNum (strict)"() -> ("Value"=w1330:dbl)  [unwired: 2 in, 2 out]
        n84 = property on="Joint3" class="DigNum (strict)"() -> ("Value"=w1329:dbl)  [unwired: 2 in, 2 out]
        n85 = property on="Increment(0-10mm)" class="DigNum (strict)"() -> ("Value"=w1327:dbl)  [unwired: 2 in, 2 out]
        n86 = Build Array(w1331, w1330, w1329) -> (w1328:dbl[])
        n87 = mathscript code="l1=110;\nl2=220;\nl3=250;\nq=q./180*pi;\nth1=q(1);\nth2=q(2);\nth3=q(3);\nT=1;\nxs=[cos(th1)*(l1 + l3*cos(th3) + l2*cos(th2)),sin(th1)*(l1 + l3*cos(th3) + l2*cos(th2)),l3*sin(th3) + l2*sin(th2)]';\nxe=xs+[-inc;0;0];\nx=xe(1);\ny=xe(2);\nz=xe(3);\nq_new(1)=atan2(y,x);\nr=sqrt(x^2+y^2)-l1;\ndq=acos((r^2+z^2-l2^2-l3^2)/(2*l2*l3));\nm=(r^2+z^2+l3^2-l2^2)/(2*l3);\nfy=atan2(r,z);\nq_new(3)=asin(m/sqrt(r^2+z^2))-fy;\nq_new(2)=q_new(3)+dq;\nfor i=1:3\na(i)=(2*q(i))/T^3 - (2*q_new(i))/T^3;\nb(i)=(3*q_new(i))/T^2 - (3*q(i))/T^2;\nd(i)=q(i);\nend\nfor j=1:3\nfor i=0:10\n vel_q(j,i+1)=3*a(j)*(0.1*i)^2+2*b(j)*0.1*i;\nend\nend\nf=vel_q./pi*32000;"("q"=w1328, "inc"=w1327) -> ("f"=w1326:cdb[][])  [unwired: 1 in, 1 out]
        n88 = Complex To Re/Im(x + iy=w1326) -> (x=w1325:dbl[][])  [unwired: 1 out]
        n89 = node-c288() -> (w1333:T1)  [unwired: 4 in]
        n90 = timed-loop {
          timing: w1333 -> [_]
          timing-out: [_] -> w1332
          tunnel: w1325 -> [w1338]
          i -> [w1342]
          stop <- w1339 stop-if-true
          n91 = node-c288() -> ()  [unwired: 1 in, 1 out]
          n92 = Index Array(array=w1338, index (col)=w1342) -> (element=w1337:dbl[])  [unwired: 1 in]
          n93 = Greater?(x=w1342, y=11) -> (0:w1340:bool)
          n94 = case shown="True" w1340 {
            tunnel: [_ TRUE] -> w1339
            frame False {
            }
            frame True {
              n95 = property on="Duty cycle3" class="DigNum (strict)"("Value"=0.0 ("Duty cycle3")) -> ()  [unwired: 2 in, 2 out]
              n96 = property on="Duty cycle2" class="DigNum (strict)"("Value"=0.0 ("Duty cycle2")) -> ()  [unwired: 2 in, 2 out]
              n97 = property on="Duty cycle1" class="DigNum (strict)"("Value"=0.0 ("Duty cycle1")) -> ()  [unwired: 2 in, 2 out]
            }
          }
          n98 = Index Array(array=w1337, index #1=0 ("index"), index #2=1 ("index"), index #3=2 ("index")) -> (element #1=w1336:dbl, element #2=w1335:dbl, element #3=w1334:dbl)
          n99 = Less Than 0?(x=w1336) -> (x < 0?=w1363:bool)
          n100 = Absolute Value(x=w1336) -> (abs(x)=w1354:dbl)
          n101 = Less Than 0?(x=w1335) -> (x < 0?=w1362:bool)
          n102 = Absolute Value(x=w1335) -> (abs(x)=w1348:dbl)
          n103 = Greater Than 0?(x=w1334) -> (x > 0?=w1355:bool)
          n104 = Absolute Value(x=w1334) -> (abs(x)=w1345:dbl)
          n105 = property on="DIR1" class="Bool (strict)"("Value"=w1363) -> ()  [unwired: 2 in, 2 out]
          n106 = property on="Frequency1" class="DigNum (strict)"("Value"=w1354) -> ()  [unwired: 2 in, 2 out]
          n107 = property on="DIR2" class="Bool (strict)"("Value"=w1362) -> ()  [unwired: 2 in, 2 out]
          n108 = property on="Frequency2" class="DigNum (strict)"("Value"=w1348) -> ()  [unwired: 2 in, 2 out]
          n109 = property on="DIR3" class="Bool (strict)"("Value"=w1355) -> ()  [unwired: 2 in, 2 out]
          n110 = Less?(x=w1354, y=1.0) -> (x < y?=w1352:bool)
          n111 = Less?(x=w1348, y=1.0) -> (x < y?=w1346:bool)
          n112 = Less?(x=w1345, y=1.0) -> (x < y?=w1343:bool)
          n113 = property on="Frequency3" class="DigNum (strict)"("Value"=w1345) -> ()  [unwired: 2 in, 2 out]
          n114 = Select(t=0.0, s=w1352, f=0.5) -> (s? t:f=w1349:dbl)
          n115 = Select(t=0.0, s=w1346, f=0.5) -> (s? t:f=w1361:dbl)
          n116 = Select(t=0.0, s=w1343, f=0.5) -> (s? t:f=w1356:dbl)
          n117 = property on="Duty cycle1" class="DigNum (strict)"("Value"=w1349) -> ()  [unwired: 2 in, 2 out]
          n118 = property on="Duty cycle2" class="DigNum (strict)"("Value"=w1361) -> ()  [unwired: 2 in, 2 out]
          n119 = property on="Duty cycle3" class="DigNum (strict)"("Value"=w1356) -> ()  [unwired: 2 in, 2 out]
          n120 = node-c288() -> ()  [unwired: 1 in, 1 out]
        }
        n121 = node-c288(w1332) -> ()  [unwired: 1 out]
      }
      event "Y+": Value Change {
        n122 = event-data() -> ()  [unwired: 1 in, 6 out]
        n123 = property on="Joint1" class="DigNum (strict)"() -> ("Value"=w2103:dbl)  [unwired: 2 in, 2 out]
        n124 = property on="Joint2" class="DigNum (strict)"() -> ("Value"=w2102:dbl)  [unwired: 2 in, 2 out]
        n125 = property on="Joint3" class="DigNum (strict)"() -> ("Value"=w2101:dbl)  [unwired: 2 in, 2 out]
        n126 = property on="Increment(0-10mm)" class="DigNum (strict)"() -> ("Value"=w2099:dbl)  [unwired: 2 in, 2 out]
        n127 = Build Array(w2103, w2102, w2101) -> (w2100:dbl[])
        n128 = mathscript code="l1=110;\nl2=220;\nl3=250;\nq=q./180*pi;\nth1=q(1);\nth2=q(2);\nth3=q(3);\nT=1;\nxs=[cos(th1)*(l1 + l3*cos(th3) + l2*cos(th2)),sin(th1)*(l1 + l3*cos(th3) + l2*cos(th2)),l3*sin(th3) + l2*sin(th2)]';\nxe=xs+[0;inc;0];\nx=xe(1);\ny=xe(2);\nz=xe(3);\nq_new(1)=atan2(y,x);\nr=sqrt(x^2+y^2)-l1;\ndq=acos((r^2+z^2-l2^2-l3^2)/(2*l2*l3));\nm=(r^2+z^2+l3^2-l2^2)/(2*l3);\nfy=atan2(r,z);\nq_new(3)=asin(m/sqrt(r^2+z^2))-fy;\nq_new(2)=q_new(3)+dq;\nfor i=1:3\na(i)=(2*q(i))/T^3 - (2*q_new(i))/T^3;\nb(i)=(3*q_new(i))/T^2 - (3*q(i))/T^2;\nd(i)=q(i);\nend\nfor j=1:3\nfor i=0:10\n vel_q(j,i+1)=3*a(j)*(0.1*i)^2+2*b(j)*0.1*i;\nend\nend\nf=vel_q./pi*32000;"("q"=w2100, "inc"=w2099) -> ("f"=w2098:cdb[][])  [unwired: 1 in, 1 out]
        n129 = Complex To Re/Im(x + iy=w2098) -> (x=w2097:dbl[][])  [unwired: 1 out]
        n130 = node-c288() -> (w2105:T1)  [unwired: 4 in]
        n131 = timed-loop {
          timing: w2105 -> [_]
          timing-out: [_] -> w2104
          tunnel: w2097 -> [w2110]
          i -> [w2114]
          stop <- w2111 stop-if-true
          n132 = node-c288() -> ()  [unwired: 1 in, 1 out]
          n133 = Index Array(array=w2110, index (col)=w2114) -> (element=w2109:dbl[])  [unwired: 1 in]
          n134 = Greater?(x=w2114, y=11) -> (0:w2112:bool)
          n135 = case shown="True" w2112 {
            tunnel: [_ TRUE] -> w2111
            frame False {
            }
            frame True {
              n136 = property on="Duty cycle3" class="DigNum (strict)"("Value"=0.0 ("Duty cycle3")) -> ()  [unwired: 2 in, 2 out]
              n137 = property on="Duty cycle2" class="DigNum (strict)"("Value"=0.0 ("Duty cycle2")) -> ()  [unwired: 2 in, 2 out]
              n138 = property on="Duty cycle1" class="DigNum (strict)"("Value"=0.0 ("Duty cycle1")) -> ()  [unwired: 2 in, 2 out]
            }
          }
          n139 = Index Array(array=w2109, index #1=0 ("index"), index #2=1 ("index"), index #3=2 ("index")) -> (element #1=w2108:dbl, element #2=w2107:dbl, element #3=w2106:dbl)
          n140 = Less Than 0?(x=w2108) -> (x < 0?=w2135:bool)
          n141 = Absolute Value(x=w2108) -> (abs(x)=w2126:dbl)
          n142 = Less Than 0?(x=w2107) -> (x < 0?=w2134:bool)
          n143 = Absolute Value(x=w2107) -> (abs(x)=w2120:dbl)
          n144 = Greater Than 0?(x=w2106) -> (x > 0?=w2127:bool)
          n145 = Absolute Value(x=w2106) -> (abs(x)=w2117:dbl)
          n146 = property on="DIR1" class="Bool (strict)"("Value"=w2135) -> ()  [unwired: 2 in, 2 out]
          n147 = property on="Frequency1" class="DigNum (strict)"("Value"=w2126) -> ()  [unwired: 2 in, 2 out]
          n148 = property on="DIR2" class="Bool (strict)"("Value"=w2134) -> ()  [unwired: 2 in, 2 out]
          n149 = property on="Frequency2" class="DigNum (strict)"("Value"=w2120) -> ()  [unwired: 2 in, 2 out]
          n150 = property on="DIR3" class="Bool (strict)"("Value"=w2127) -> ()  [unwired: 2 in, 2 out]
          n151 = Less?(x=w2126, y=1.0) -> (x < y?=w2124:bool)
          n152 = Less?(x=w2120, y=1.0) -> (x < y?=w2118:bool)
          n153 = Less?(x=w2117, y=1.0) -> (x < y?=w2115:bool)
          n154 = property on="Frequency3" class="DigNum (strict)"("Value"=w2117) -> ()  [unwired: 2 in, 2 out]
          n155 = Select(t=0.0, s=w2124, f=0.5) -> (s? t:f=w2121:dbl)
          n156 = Select(t=0.0, s=w2118, f=0.5) -> (s? t:f=w2133:dbl)
          n157 = Select(t=0.0, s=w2115, f=0.5) -> (s? t:f=w2128:dbl)
          n158 = property on="Duty cycle1" class="DigNum (strict)"("Value"=w2121) -> ()  [unwired: 2 in, 2 out]
          n159 = property on="Duty cycle2" class="DigNum (strict)"("Value"=w2133) -> ()  [unwired: 2 in, 2 out]
          n160 = property on="Duty cycle3" class="DigNum (strict)"("Value"=w2128) -> ()  [unwired: 2 in, 2 out]
          n161 = node-c288() -> ()  [unwired: 1 in, 1 out]
        }
        n162 = node-c288(w2104) -> ()  [unwired: 1 out]
      }
      event "Y-": Value Change {
        n163 = event-data() -> ()  [unwired: 1 in, 6 out]
        n164 = property on="Joint1" class="DigNum (strict)"() -> ("Value"=w2873:dbl)  [unwired: 2 in, 2 out]
        n165 = property on="Joint2" class="DigNum (strict)"() -> ("Value"=w2872:dbl)  [unwired: 2 in, 2 out]
        n166 = property on="Joint3" class="DigNum (strict)"() -> ("Value"=w2871:dbl)  [unwired: 2 in, 2 out]
        n167 = property on="Increment(0-10mm)" class="DigNum (strict)"() -> ("Value"=w2869:dbl)  [unwired: 2 in, 2 out]
        n168 = Build Array(w2873, w2872, w2871) -> (w2870:dbl[])
        n169 = mathscript code="l1=110;\nl2=220;\nl3=250;\nq=q./180*pi;\nth1=q(1);\nth2=q(2);\nth3=q(3);\nT=1;\nxs=[cos(th1)*(l1 + l3*cos(th3) + l2*cos(th2)),sin(th1)*(l1 + l3*cos(th3) + l2*cos(th2)),l3*sin(th3) + l2*sin(th2)]';\nxe=xs+[0;-inc;0];\nx=xe(1);\ny=xe(2);\nz=xe(3);\nq_new(1)=atan2(y,x);\nr=sqrt(x^2+y^2)-l1;\ndq=acos((r^2+z^2-l2^2-l3^2)/(2*l2*l3));\nm=(r^2+z^2+l3^2-l2^2)/(2*l3);\nfy=atan2(r,z);\nq_new(3)=asin(m/sqrt(r^2+z^2))-fy;\nq_new(2)=q_new(3)+dq;\nfor i=1:3\na(i)=(2*q(i))/T^3 - (2*q_new(i))/T^3;\nb(i)=(3*q_new(i))/T^2 - (3*q(i))/T^2;\nd(i)=q(i);\nend\nfor j=1:3\nfor i=0:10\n vel_q(j,i+1)=3*a(j)*(0.1*i)^2+2*b(j)*0.1*i;\nend\nend\nf=vel_q./pi*32000;"("q"=w2870, "inc"=w2869) -> ("f"=w2868:cdb[][])  [unwired: 1 in, 1 out]
        n170 = Complex To Re/Im(x + iy=w2868) -> (x=w2867:dbl[][])  [unwired: 1 out]
        n171 = node-c288() -> (w2875:T1)  [unwired: 4 in]
        n172 = timed-loop {
          timing: w2875 -> [_]
          timing-out: [_] -> w2874
          tunnel: w2867 -> [w2880]
          i -> [w2884]
          stop <- w2881 stop-if-true
          n173 = node-c288() -> ()  [unwired: 1 in, 1 out]
          n174 = Index Array(array=w2880, index (col)=w2884) -> (element=w2879:dbl[])  [unwired: 1 in]
          n175 = Greater?(x=w2884, y=11) -> (0:w2882:bool)
          n176 = case shown="True" w2882 {
            tunnel: [_ TRUE] -> w2881
            frame False {
            }
            frame True {
              n177 = property on="Duty cycle3" class="DigNum (strict)"("Value"=0.0 ("Duty cycle3")) -> ()  [unwired: 2 in, 2 out]
              n178 = property on="Duty cycle2" class="DigNum (strict)"("Value"=0.0 ("Duty cycle2")) -> ()  [unwired: 2 in, 2 out]
              n179 = property on="Duty cycle1" class="DigNum (strict)"("Value"=0.0 ("Duty cycle1")) -> ()  [unwired: 2 in, 2 out]
            }
          }
          n180 = Index Array(array=w2879, index #1=0 ("index"), index #2=1 ("index"), index #3=2 ("index")) -> (element #1=w2878:dbl, element #2=w2877:dbl, element #3=w2876:dbl)
          n181 = Less Than 0?(x=w2878) -> (x < 0?=w2905:bool)
          n182 = Absolute Value(x=w2878) -> (abs(x)=w2896:dbl)
          n183 = Less Than 0?(x=w2877) -> (x < 0?=w2904:bool)
          n184 = Absolute Value(x=w2877) -> (abs(x)=w2890:dbl)
          n185 = Greater Than 0?(x=w2876) -> (x > 0?=w2897:bool)
          n186 = Absolute Value(x=w2876) -> (abs(x)=w2887:dbl)
          n187 = property on="DIR1" class="Bool (strict)"("Value"=w2905) -> ()  [unwired: 2 in, 2 out]
          n188 = property on="Frequency1" class="DigNum (strict)"("Value"=w2896) -> ()  [unwired: 2 in, 2 out]
          n189 = property on="DIR2" class="Bool (strict)"("Value"=w2904) -> ()  [unwired: 2 in, 2 out]
          n190 = property on="Frequency2" class="DigNum (strict)"("Value"=w2890) -> ()  [unwired: 2 in, 2 out]
          n191 = property on="DIR3" class="Bool (strict)"("Value"=w2897) -> ()  [unwired: 2 in, 2 out]
          n192 = Less?(x=w2896, y=1.0) -> (x < y?=w2894:bool)
          n193 = Less?(x=w2890, y=1.0) -> (x < y?=w2888:bool)
          n194 = Less?(x=w2887, y=1.0) -> (x < y?=w2885:bool)
          n195 = property on="Frequency3" class="DigNum (strict)"("Value"=w2887) -> ()  [unwired: 2 in, 2 out]
          n196 = Select(t=0.0, s=w2894, f=0.5) -> (s? t:f=w2891:dbl)
          n197 = Select(t=0.0, s=w2888, f=0.5) -> (s? t:f=w2903:dbl)
          n198 = Select(t=0.0, s=w2885, f=0.5) -> (s? t:f=w2898:dbl)
          n199 = property on="Duty cycle1" class="DigNum (strict)"("Value"=w2891) -> ()  [unwired: 2 in, 2 out]
          n200 = property on="Duty cycle2" class="DigNum (strict)"("Value"=w2903) -> ()  [unwired: 2 in, 2 out]
          n201 = property on="Duty cycle3" class="DigNum (strict)"("Value"=w2898) -> ()  [unwired: 2 in, 2 out]
          n202 = node-c288() -> ()  [unwired: 1 in, 1 out]
        }
        n203 = node-c288(w2874) -> ()  [unwired: 1 out]
      }
      event "Z+": Value Change {
        n204 = event-data() -> ()  [unwired: 1 in, 6 out]
        n205 = property on="Joint1" class="DigNum (strict)"() -> ("Value"=w3645:dbl)  [unwired: 2 in, 2 out]
        n206 = property on="Joint2" class="DigNum (strict)"() -> ("Value"=w3644:dbl)  [unwired: 2 in, 2 out]
        n207 = property on="Joint3" class="DigNum (strict)"() -> ("Value"=w3643:dbl)  [unwired: 2 in, 2 out]
        n208 = property on="Increment(0-10mm)" class="DigNum (strict)"() -> ("Value"=w3641:dbl)  [unwired: 2 in, 2 out]
        n209 = Build Array(w3645, w3644, w3643) -> (w3642:dbl[])
        n210 = mathscript code="l1=110;\nl2=220;\nl3=250;\nq=q./180*pi;\nth1=q(1);\nth2=q(2);\nth3=q(3);\nT=1;\nxs=[cos(th1)*(l1 + l3*cos(th3) + l2*cos(th2)),sin(th1)*(l1 + l3*cos(th3) + l2*cos(th2)),l3*sin(th3) + l2*sin(th2)]';\nxe=xs+[0;0;inc];\nx=xe(1);\ny=xe(2);\nz=xe(3);\nq_new(1)=atan2(y,x);\nr=sqrt(x^2+y^2)-l1;\ndq=acos((r^2+z^2-l2^2-l3^2)/(2*l2*l3));\nm=(r^2+z^2+l3^2-l2^2)/(2*l3);\nfy=atan2(r,z);\nq_new(3)=asin(m/sqrt(r^2+z^2))-fy;\nq_new(2)=q_new(3)+dq;\nfor i=1:3\na(i)=(2*q(i))/T^3 - (2*q_new(i))/T^3;\nb(i)=(3*q_new(i))/T^2 - (3*q(i))/T^2;\nd(i)=q(i);\nend\nfor j=1:3\nfor i=0:10\n vel_q(j,i+1)=3*a(j)*(0.1*i)^2+2*b(j)*0.1*i;\nend\nend\nf=vel_q./pi*32000;"("q"=w3642, "inc"=w3641) -> ("f"=w3640:cdb[][])  [unwired: 1 in, 1 out]
        n211 = Complex To Re/Im(x + iy=w3640) -> (x=w3639:dbl[][])  [unwired: 1 out]
        n212 = node-c288() -> (w3647:T1)  [unwired: 4 in]
        n213 = timed-loop {
          timing: w3647 -> [_]
          timing-out: [_] -> w3646
          tunnel: w3639 -> [w3652]
          i -> [w3656]
          stop <- w3653 stop-if-true
          n214 = node-c288() -> ()  [unwired: 1 in, 1 out]
          n215 = Index Array(array=w3652, index (col)=w3656) -> (element=w3651:dbl[])  [unwired: 1 in]
          n216 = Greater?(x=w3656, y=11) -> (0:w3654:bool)
          n217 = case shown="True" w3654 {
            tunnel: [_ TRUE] -> w3653
            frame False {
            }
            frame True {
              n218 = property on="Duty cycle3" class="DigNum (strict)"("Value"=0.0 ("Duty cycle3")) -> ()  [unwired: 2 in, 2 out]
              n219 = property on="Duty cycle2" class="DigNum (strict)"("Value"=0.0 ("Duty cycle2")) -> ()  [unwired: 2 in, 2 out]
              n220 = property on="Duty cycle1" class="DigNum (strict)"("Value"=0.0 ("Duty cycle1")) -> ()  [unwired: 2 in, 2 out]
            }
          }
          n221 = Index Array(array=w3651, index #1=0 ("index"), index #2=1 ("index"), index #3=2 ("index")) -> (element #1=w3650:dbl, element #2=w3649:dbl, element #3=w3648:dbl)
          n222 = Less Than 0?(x=w3650) -> (x < 0?=w3677:bool)
          n223 = Absolute Value(x=w3650) -> (abs(x)=w3668:dbl)
          n224 = Less Than 0?(x=w3649) -> (x < 0?=w3676:bool)
          n225 = Absolute Value(x=w3649) -> (abs(x)=w3662:dbl)
          n226 = Greater Than 0?(x=w3648) -> (x > 0?=w3669:bool)
          n227 = Absolute Value(x=w3648) -> (abs(x)=w3659:dbl)
          n228 = property on="DIR1" class="Bool (strict)"("Value"=w3677) -> ()  [unwired: 2 in, 2 out]
          n229 = property on="Frequency1" class="DigNum (strict)"("Value"=w3668) -> ()  [unwired: 2 in, 2 out]
          n230 = property on="DIR2" class="Bool (strict)"("Value"=w3676) -> ()  [unwired: 2 in, 2 out]
          n231 = property on="Frequency2" class="DigNum (strict)"("Value"=w3662) -> ()  [unwired: 2 in, 2 out]
          n232 = property on="DIR3" class="Bool (strict)"("Value"=w3669) -> ()  [unwired: 2 in, 2 out]
          n233 = Less?(x=w3668, y=1.0) -> (x < y?=w3666:bool)
          n234 = Less?(x=w3662, y=1.0) -> (x < y?=w3660:bool)
          n235 = Less?(x=w3659, y=1.0) -> (x < y?=w3657:bool)
          n236 = property on="Frequency3" class="DigNum (strict)"("Value"=w3659) -> ()  [unwired: 2 in, 2 out]
          n237 = Select(t=0.0, s=w3666, f=0.5) -> (s? t:f=w3663:dbl)
          n238 = Select(t=0.0, s=w3660, f=0.5) -> (s? t:f=w3675:dbl)
          n239 = Select(t=0.0, s=w3657, f=0.5) -> (s? t:f=w3670:dbl)
          n240 = property on="Duty cycle1" class="DigNum (strict)"("Value"=w3663) -> ()  [unwired: 2 in, 2 out]
          n241 = property on="Duty cycle2" class="DigNum (strict)"("Value"=w3675) -> ()  [unwired: 2 in, 2 out]
          n242 = property on="Duty cycle3" class="DigNum (strict)"("Value"=w3670) -> ()  [unwired: 2 in, 2 out]
          n243 = node-c288() -> ()  [unwired: 1 in, 1 out]
        }
        n244 = node-c288(w3646) -> ()  [unwired: 1 out]
      }
      event "Z-": Value Change {
        n245 = event-data() -> ()  [unwired: 1 in, 6 out]
        n246 = property on="Joint1" class="DigNum (strict)"() -> ("Value"=w4415:dbl)  [unwired: 2 in, 2 out]
        n247 = property on="Joint2" class="DigNum (strict)"() -> ("Value"=w4414:dbl)  [unwired: 2 in, 2 out]
        n248 = property on="Joint3" class="DigNum (strict)"() -> ("Value"=w4413:dbl)  [unwired: 2 in, 2 out]
        n249 = property on="Increment(0-10mm)" class="DigNum (strict)"() -> ("Value"=w4411:dbl)  [unwired: 2 in, 2 out]
        n250 = Build Array(w4415, w4414, w4413) -> (w4412:dbl[])
        n251 = mathscript code="l1=110;\nl2=220;\nl3=250;\nq=q./180*pi;\nth1=q(1);\nth2=q(2);\nth3=q(3);\nT=1;\nxs=[cos(th1)*(l1 + l3*cos(th3) + l2*cos(th2)),sin(th1)*(l1 + l3*cos(th3) + l2*cos(th2)),l3*sin(th3) + l2*sin(th2)]';\nxe=xs+[0;0;-inc];\nx=xe(1);\ny=xe(2);\nz=xe(3);\nq_new(1)=atan2(y,x);\nr=sqrt(x^2+y^2)-l1;\ndq=acos((r^2+z^2-l2^2-l3^2)/(2*l2*l3));\nm=(r^2+z^2+l3^2-l2^2)/(2*l3);\nfy=atan2(r,z);\nq_new(3)=asin(m/sqrt(r^2+z^2))-fy;\nq_new(2)=q_new(3)+dq;\nfor i=1:3\na(i)=(2*q(i))/T^3 - (2*q_new(i))/T^3;\nb(i)=(3*q_new(i))/T^2 - (3*q(i))/T^2;\nd(i)=q(i);\nend\nfor j=1:3\nfor i=0:10\n vel_q(j,i+1)=3*a(j)*(0.1*i)^2+2*b(j)*0.1*i;\nend\nend\nf=vel_q./pi*32000;"("q"=w4412, "inc"=w4411) -> ("f"=w4410:cdb[][])  [unwired: 1 in, 1 out]
        n252 = Complex To Re/Im(x + iy=w4410) -> (x=w4409:dbl[][])  [unwired: 1 out]
        n253 = node-c288() -> (w4417:T1)  [unwired: 4 in]
        n254 = timed-loop {
          timing: w4417 -> [_]
          timing-out: [_] -> w4416
          tunnel: w4409 -> [w4422]
          i -> [w4426]
          stop <- w4423 stop-if-true
          n255 = node-c288() -> ()  [unwired: 1 in, 1 out]
          n256 = Index Array(array=w4422, index (col)=w4426) -> (element=w4421:dbl[])  [unwired: 1 in]
          n257 = Greater?(x=w4426, y=11) -> (0:w4424:bool)
          n258 = case shown="True" w4424 {
            tunnel: [_ TRUE] -> w4423
            frame False {
            }
            frame True {
              n259 = property on="Duty cycle3" class="DigNum (strict)"("Value"=0.0 ("Duty cycle3")) -> ()  [unwired: 2 in, 2 out]
              n260 = property on="Duty cycle2" class="DigNum (strict)"("Value"=0.0 ("Duty cycle2")) -> ()  [unwired: 2 in, 2 out]
              n261 = property on="Duty cycle1" class="DigNum (strict)"("Value"=0.0 ("Duty cycle1")) -> ()  [unwired: 2 in, 2 out]
            }
          }
          n262 = Index Array(array=w4421, index #1=0 ("index"), index #2=1 ("index"), index #3=2 ("index")) -> (element #1=w4420:dbl, element #2=w4419:dbl, element #3=w4418:dbl)
          n263 = Less Than 0?(x=w4420) -> (x < 0?=w4447:bool)
          n264 = Absolute Value(x=w4420) -> (abs(x)=w4438:dbl)
          n265 = Less Than 0?(x=w4419) -> (x < 0?=w4446:bool)
          n266 = Absolute Value(x=w4419) -> (abs(x)=w4432:dbl)
          n267 = Greater Than 0?(x=w4418) -> (x > 0?=w4439:bool)
          n268 = Absolute Value(x=w4418) -> (abs(x)=w4429:dbl)
          n269 = property on="DIR1" class="Bool (strict)"("Value"=w4447) -> ()  [unwired: 2 in, 2 out]
          n270 = property on="Frequency1" class="DigNum (strict)"("Value"=w4438) -> ()  [unwired: 2 in, 2 out]
          n271 = property on="DIR2" class="Bool (strict)"("Value"=w4446) -> ()  [unwired: 2 in, 2 out]
          n272 = property on="Frequency2" class="DigNum (strict)"("Value"=w4432) -> ()  [unwired: 2 in, 2 out]
          n273 = property on="DIR3" class="Bool (strict)"("Value"=w4439) -> ()  [unwired: 2 in, 2 out]
          n274 = Less?(x=w4438, y=1.0) -> (x < y?=w4436:bool)
          n275 = Less?(x=w4432, y=1.0) -> (x < y?=w4430:bool)
          n276 = Less?(x=w4429, y=1.0) -> (x < y?=w4427:bool)
          n277 = property on="Frequency3" class="DigNum (strict)"("Value"=w4429) -> ()  [unwired: 2 in, 2 out]
          n278 = Select(t=0.0, s=w4436, f=0.5) -> (s? t:f=w4433:dbl)
          n279 = Select(t=0.0, s=w4430, f=0.5) -> (s? t:f=w4445:dbl)
          n280 = Select(t=0.0, s=w4427, f=0.5) -> (s? t:f=w4440:dbl)
          n281 = property on="Duty cycle1" class="DigNum (strict)"("Value"=w4433) -> ()  [unwired: 2 in, 2 out]
          n282 = property on="Duty cycle2" class="DigNum (strict)"("Value"=w4445) -> ()  [unwired: 2 in, 2 out]
          n283 = property on="Duty cycle3" class="DigNum (strict)"("Value"=w4440) -> ()  [unwired: 2 in, 2 out]
          n284 = node-c288() -> ()  [unwired: 1 in, 1 out]
        }
        n285 = node-c288(w4416) -> ()  [unwired: 1 out]
      }
      event "Circle": Value Change {
        n286 = event-data() -> ()  [unwired: 1 in, 6 out]
        n287 = node-c288() -> (w5186:T1)  [unwired: 5 in]
        n288 = timed-loop {
          timing: w5186 -> [_]
          timing-out: [_] -> w5185
          i -> [w5189]
          stop <- w5187 stop-if-true
          n289 = node-c288() -> ()  [unwired: 1 in, 1 out]
          n290 = mathscript code="l1=110;\nl2=220;\nl3=250;\nt=0.1*i;\nXC=[455 0 220]';\nr=15;\nP=XC+[r*cos(pi*t),r*sin(pi*t),0]';\nPd=[-r*pi*sin(pi*t);r*pi*cos(pi*t);0];\nx=P(1);\ny=P(2);\nz=P(3);\nq(1)=atan2(y,x);\nr=sqrt(x^2+y^2)-l1;\ndq=acos((r^2+z^2-l2^2-l3^2)/(2*l2*l3));\nm=(r^2+z^2+l3^2-l2^2)/(2*l3);\nfy=atan2(r,z);\nq(3)=asin(m/sqrt(r^2+z^2))-fy;\nq(2)=q(3)+dq;\nth1=q(1);\nth2=q(2);\nth3=q(3);\nJ=[ -sin(th1)*(l1 + l2*cos(th2) + l3*cos(th3)), -l2*cos(th1)*sin(th2), -l3*cos(th1)*sin(th3)\n  cos(th1)*(l1 + l2*cos(th2) + l3*cos(th3)), -l2*sin(th1)*sin(th2), -l3*sin(th1)*sin(th3)\n                                          0,           l2*cos(th2),           l3*cos(th3)];\nqd=pinv(J)*Pd;\nf=qd./pi*32000;\nf=f(:,1);"("i"=w5189) -> ("f"=w5218:cdb[])  [unwired: 1 in, 1 out]
          n291 = Equal?(x=w5189, y=20) -> (x = y?=w5187:bool)
          n292 = Complex To Re/Im(x + iy=w5218) -> (x=w5217:dbl[])  [unwired: 1 out]
          "circle" <- w5217
          n293 = Index Array(array=w5217, index #1=0 ("index"), index #2=1 ("index"), index #3=2 ("index")) -> (element #1=w5215:dbl, element #2=w5210:dbl, element #3=w5209:dbl)
          n294 = Less Than 0?(x=w5215) -> (x < 0?=w5216:bool)
          n295 = Absolute Value(x=w5215) -> (abs(x)=w5208:dbl)
          n296 = Less Than 0?(x=w5210) -> (x < 0?=w5214:bool)
          n297 = Absolute Value(x=w5210) -> (abs(x)=w5205:dbl)
          n298 = Greater Than 0?(x=w5209) -> (x > 0?=w5211:bool)
          n299 = Absolute Value(x=w5209) -> (abs(x)=w5203:dbl)
          n300 = property on="Frequency2" class="DigNum (strict)"("Value"=w5205) -> ()  [unwired: 2 in, 2 out]
          n301 = Less?(x=w5208, y=10.0) -> (x < y?=w5207:bool)
          n302 = Less?(x=w5205, y=10.0) -> (x < y?=w5204:bool)
          n303 = Less?(x=w5203, y=10.0) -> (x < y?=w5202:bool)
          n304 = Select(t=0.0, s=w5207, f=0.5) -> (s? t:f=w5206:dbl)
          n305 = Select(t=0.0, s=w5204, f=0.5) -> (s? t:f=w5213:dbl)
          n306 = Select(t=0.0, s=w5202, f=0.5) -> (s? t:f=w5212:dbl)
          n307 = property on="DIR1" class="Bool (strict)"("Value"=w5216) -> ()  [unwired: 2 in, 2 out]
          n308 = property on="Duty cycle1" class="DigNum (strict)"("Value"=w5206) -> ()  [unwired: 2 in, 2 out]
          n309 = property on="Duty cycle2" class="DigNum (strict)"("Value"=w5213) -> ()  [unwired: 2 in, 2 out]
          n310 = property on="Duty cycle3" class="DigNum (strict)"("Value"=w5212) -> ()  [unwired: 2 in, 2 out]
          n311 = property on="DIR2" class="Bool (strict)"("Value"=w5214) -> ()  [unwired: 2 in, 2 out]
          n312 = property on="Frequency3" class="DigNum (strict)"("Value"=w5203) -> ()  [unwired: 2 in, 2 out]
          n313 = property on="Frequency1" class="DigNum (strict)"("Value"=w5208) -> ()  [unwired: 2 in, 2 out]
          n314 = property on="DIR3" class="Bool (strict)"("Value"=w5211) -> ()  [unwired: 2 in, 2 out]
          n315 = node-c288() -> ()  [unwired: 1 in, 1 out]
        }
        n316 = node-c288(w5185) -> (w5181:errorcluster)
        n317 = property on="Duty cycle1" class="DigNum (strict)"(error in=w5181, "Value"=0.0 ("Duty cycle1")) -> ()  [unwired: 1 in, 2 out]
        n318 = property on="Duty cycle2" class="DigNum (strict)"(error in=w5181, "Value"=0.0 ("Duty cycle2")) -> ()  [unwired: 1 in, 2 out]
        n319 = property on="Duty cycle3" class="DigNum (strict)"(error in=w5181, "Value"=0.0 ("Duty cycle3")) -> ()  [unwired: 1 in, 2 out]
      }
    }
  }
